vi "CSS grouping with LCS.vi"() -> ()   [LabVIEW 2014]
uses:
  <vilib>/Utility/file.llb/Read From Spreadsheet File (string).vi
  <vilib>/Utility/file.llb/Write To Spreadsheet File (string).vi
panel:
  in  "16 groups":string[][](array[string])=array2000x3[6000 elements]
  in  "8 groups":string[][](array[string])=[["0 1 0 1 0 3 0", "10", "1"], ["0 -1 1 0 1 0 3 0", "10", "1"], ["0 1 -1 0 1 0 3 0", "10", "1"], ["0 -4 1 0 1 0 3 0", "10", "1"], ["0 1 -4 0 1 0 3 0", "10", "1"], ["0 1 0 -1 1 0 3 0", "10", "1"], ["0 -1 1 0 -1 1 0 3 0", "10", "1"], ["0 1 -1 0 -1 1 0 3 0", "10", "1"], ["0 -4 1 0 -1 1 0 3 0", "10", "1"], ["0 1 -4 0 -1 1 0 3 0", "10", "1"], ["0 1 0 1 -1 0 3 0", "10", "1"], ["0 -1 1 0 1 -1 0 3 0", "10", "1"], ["0 1 -1 0 1 -1 0 3 0", "10", "1"], ["0 -4 1 0 1 -1 0 3 0", "10", "1"], ["0 1 -4 0 1 -1 0 3 0", "10", "1"], ["0 1 0 -4 1 0 3 0", "10", "1"], ["0 -1 1 0 -4 1 0 3 0", "10", "1"], ["0 1 -1 0 -4 1 0 3 0", "10", "1"], ["0 -4 1 0 -4 1 0 3 0", "10", "1"], ["0 1 -4 0 -4 1 0 3 0", "10", "1"], ["0 1 0 1 -4 0 3 0", "10", "1"], ["0 -1 1 0 1 -4 0 3 0", "10", "1"], ["0 1 -1 0 1 -4 0 3 0", "10", "1"], ["0 -4 1 0 1 -4 0 3 0", "10", "1"], ["0 1 -4 0 1 -4 0 3 0", "10", "1"], ["0 1 0 1 0 -2 3 0", "10", "1"], ["0 -1 1 0 1 0 -2 3 0", "10", "1"], ["0 1 -1 0 1 0 -2 3 0", "10", "1"], ["0 -4 1 0 1 0 -2 3 0", "10", "1"], ["0 1 -4 0 1 0 -2 3 0", "10", "1"], ["0 1 0 -1 1 0 -2 3 0", "10", "1"], ["0 -1 1 0 -1 1 0 -2 3 0", "10", "1"], ["0 1 -1 0 -1 1 0 -2 3 0", "10", "1"], ["0 -4 1 0 -1 1 0 -2 3 0", "10", "1"], ["0 1 -4 0 -1 1 0 -2 3 0", "10", "1"], ["0 1 0 1 -1 0 -2 3 0", "10", "1"], ["0 -1 1 0 1 -1 0 -2 3 0", "10", "1"], ["0 1 -1 0 1 -1 0 -2 3 0", "10", "1"], ["0 -4 1 0 1 -1 0 -2 3 0", "10", "1"], ["0 1 -4 0 1 -1 0 -2 3 0", "10", "1"], ["0 1 0 -4 1 0 -2 3 0", "10", "1"], ["0 -1 1 0 -4 1 0 -2 3 0", "10", "1"], ["0 1 -1 0 -4 1 0 -2 3 0", "10", "1"], ["0 -4 1 0 -4 1 0 -2 3 0", "10", "1"], ["0 1 -4 0 -4 1 0 -2 3 0", "10", "1"], ["0 1 0 1 -4 0 -2 3 0", "10", "1"], ["0 -1 1 0 1 -4 0 -2 3 0", "10", "1"], ["0 1 -1 0 1 -4 0 -2 3 0", "10", "1"], ["0 -4 1 0 1 -4 0 -2 3 0", "10", "1"], ["0 1 -4 0 1 -4 0 -2 3 0", "10", "1"], ["0 1 0 1 0 3 -2 0", "10", "1"], ["0 -1 1 0 1 0 3 -2 0", "10", "1"], ["0 1 -1 0 1 0 3 -2 0", "10", "1"], ["0 -4 1 0 1 0 3 -2 0", "10", "1"], ["0 1 -4 0 1 0 3 -2 0", "10", "1"], ["0 1 0 -1 1 0 3 -2 0", "10", "1"], ["0 -1 1 0 -1 1 0 3 -2 0", "10", "1"], ["0 1 -1 0 -1 1 0 3 -2 0", "10", "1"], ["0 -4 1 0 -1 1 0 3 -2 0", "10", "1"], ["0 1 -4 0 -1 1 0 3 -2 0", "10", "1"], ["0 1 0 1 -1 0 3 -2 0", "10", "1"], ["0 -1 1 0 1 -1 0 3 -2 0", "10", "1"], ["0 1 -1 0 1 -1 0 3 -2 0", "10", "1"], ["0 -4 1 0 1 -1 0 3 -2 0", "10", "1"], ["0 1 -4 0 1 -1 0 3 -2 0", "10", "1"], ["0 1 0 -4 1 0 3 -2 0", "10", "1"], ["0 -1 1 0 -4 1 0 3 -2 0", "10", "1"], ["0 1 -1 0 -4 1 0 3 -2 0", "10", "1"], ["0 -4 1 0 -4 1 0 3 -2 0", "10", "1"], ["0 1 -4 0 -4 1 0 3 -2 0", "10", "1"], ["0 1 0 1 -4 0 3 -2 0", "10", "1"], ["0 -1 1 0 1 -4 0 3 -2 0", "10", "1"], ["0 1 -1 0 1 -4 0 3 -2 0", "10", "1"], ["0 -4 1 0 1 -4 0 3 -2 0", "10", "1"], ["0 1 -4 0 1 -4 0 3 -2 0", "10", "1"], ["0 1 0 1 0 -3 3 0", "10", "1"], ["0 -1 1 0 1 0 -3 3 0", "10", "1"], ["0 1 -1 0 1 0 -3 3 0", "10", "1"], ["0 -4 1 0 1 0 -3 3 0", "10", "1"], ["0 1 -4 0 1 0 -3 3 0", "10", "1"], ["0 1 0 -1 1 0 -3 3 0", "10", "1"], ["0 -1 1 0 -1 1 0 -3 3 0", "10", "1"], ["0 1 -1 0 -1 1 0 -3 3 0", "10", "1"], ["0 -4 1 0 -1 1 0 -3 3 0", "10", "1"], ["0 1 -4 0 -1 1 0 -3 3 0", "10", "1"], ["0 1 0 1 -1 0 -3 3 0", "10", "1"], ["0 -1 1 0 1 -1 0 -3 3 0", "10", "1"], ["0 1 -1 0 1 -1 0 -3 3 0", "10", "1"], ["0 -4 1 0 1 -1 0 -3 3 0", "10", "1"], ["0 1 -4 0 1 -1 0 -3 3 0", "10", "1"], ["0 1 0 -4 1 0 -3 3 0", "10", "1"], ["0 -1 1 0 -4 1 0 -3 3 0", "10", "1"], ["0 1 -1 0 -4 1 0 -3 3 0", "10", "1"], ["0 -4 1 0 -4 1 0 -3 3 0", "10", "1"], ["0 1 -4 0 -4 1 0 -3 3 0", "10", "1"], ["0 1 0 1 -4 0 -3 3 0", "10", "1"], ["0 -1 1 0 1 -4 0 -3 3 0", "10", "1"], ["0 1 -1 0 1 -4 0 -3 3 0", "10", "1"], ["0 -4 1 0 1 -4 0 -3 3 0", "10", "1"], ["0 1 -4 0 1 -4 0 -3 3 0", "10", "1"], ["0 1 0 1 0 3 -3 0", "10", "1"], ["0 -1 1 0 1 0 3 -3 0", "10", "1"], ["0 1 -1 0 1 0 3 -3 0", "10", "1"], ["0 -4 1 0 1 0 3 -3 0", "10", "1"], ["0 1 -4 0 1 0 3 -3 0", "10", "1"], ["0 1 0 -1 1 0 3 -3 0", "10", "1"], ["0 -1 1 0 -1 1 0 3 -3 0", "10", "1"], ["0 1 -1 0 -1 1 0 3 -3 0", "10", "1"], ["0 -4 1 0 -1 1 0 3 -3 0", "10", "1"], ["0 1 -4 0 -1 1 0 3 -3 0", "10", "1"], ["0 1 0 1 -1 0 3 -3 0", "10", "1"], ["0 -1 1 0 1 -1 0 3 -3 0", "10", "1"], ["0 1 -1 0 1 -1 0 3 -3 0", "10", "1"], ["0 -4 1 0 1 -1 0 3 -3 0", "10", "1"], ["0 1 -4 0 1 -1 0 3 -3 0", "10", "1"], ["0 1 0 -4 1 0 3 -3 0", "10", "1"], ["0 -1 1 0 -4 1 0 3 -3 0", "10", "1"], ["0 1 -1 0 -4 1 0 3 -3 0", "10", "1"], ["0 -4 1 0 -4 1 0 3 -3 0", "10", "1"], ["0 1 -4 0 -4 1 0 3 -3 0", "10", "1"], ["0 1 0 1 -4 0 3 -3 0", "10", "1"], ["0 -1 1 0 1 -4 0 3 -3 0", "10", "1"], ["0 1 -1 0 1 -4 0 3 -3 0", "10", "1"], ["0 -4 1 0 1 -4 0 3 -3 0", "10", "1"], ["0 1 -4 0 1 -4 0 3 -3 0", "10", "1"], ["0 1 0 3 0 1 0", "10", "2"], ["0 -1 1 0 3 0 1 0", "10", "2"], ["0 1 -1 0 3 0 1 0", "10", "2"], ["0 -4 1 0 3 0 1 0", "10", "2"], ["0 1 -4 0 3 0 1 0", "10", "2"], ["0 1 0 -2 3 0 1 0", "10", "2"], ["0 -1 1 0 -2 3 0 1 0", "10", "2"], ["0 1 -1 0 -2 3 0 1 0", "10", "2"], ["0 -4 1 0 -2 3 0 1 0", "10", "2"], ["0 1 -4 0 -2 3 0 1 0", "10", "2"], ["0 1 0 3 -2 0 1 0", "10", "2"], ["0 -1 1 0 3 -2 0 1 0", "10", "2"], ["0 1 -1 0 3 -2 0 1 0", "10", "2"], ["0 -4 1 0 3 -2 0 1 0", "10", "2"], ["0 1 -4 0 3 -2 0 1 0", "10", "2"], ["0 1 0 -3 3 0 1 0", "10", "2"], ["0 -1 1 0 -3 3 0 1 0", "10", "2"], ["0 1 -1 0 -3 3 0 1 0", "10", "2"], ["0 -4 1 0 -3 3 0 1 0", "10", "2"], ["0 1 -4 0 -3 3 0 1 0", "10", "2"], ["0 1 0 3 -3 0 1 0", "10", "2"], ["0 -1 1 0 3 -3 0 1 0", "10", "2"], ["0 1 -1 0 3 -3 0 1 0", "10", "2"], ["0 -4 1 0 3 -3 0 1 0", "10", "2"], ["0 1 -4 0 3 -3 0 1 0", "10", "2"], ["0 1 0 3 0 -1 1 0", "10", "2"], ["0 -1 1 0 3 0 -1 1 0", "10", "2"], ["0 1 -1 0 3 0 -1 1 0", "10", "2"], ["0 -4 1 0 3 0 -1 1 0", "10", "2"], ["0 1 -4 0 3 0 -1 1 0", "10", "2"], ["0 1 0 -2 3 0 -1 1 0", "10", "2"], ["0 -1 1 0 -2 3 0 -1 1 0", "10", "2"], ["0 1 -1 0 -2 3 0 -1 1 0", "10", "2"], ["0 -4 1 0 -2 3 0 -1 1 0", "10", "2"], ["0 1 -4 0 -2 3 0 -1 1 0", "10", "2"], ["0 1 0 3 -2 0 -1 1 0", "10", "2"], ["0 -1 1 0 3 -2 0 -1 1 0", "10", "2"], ["0 1 -1 0 3 -2 0 -1 1 0", "10", "2"], ["0 -4 1 0 3 -2 0 -1 1 0", "10", "2"], ["0 1 -4 0 3 -2 0 -1 1 0", "10", "2"], ["0 1 0 -3 3 0 -1 1 0", "10", "2"], ["0 -1 1 0 -3 3 0 -1 1 0", "10", "2"], ["0 1 -1 0 -3 3 0 -1 1 0", "10", "2"], ["0 -4 1 0 -3 3 0 -1 1 0", "10", "2"], ["0 1 -4 0 -3 3 0 -1 1 0", "10", "2"], ["0 1 0 3 -3 0 -1 1 0", "10", "2"], ["0 -1 1 0 3 -3 0 -1 1 0", "10", "2"], ["0 1 -1 0 3 -3 0 -1 1 0", "10", "2"], ["0 -4 1 0 3 -3 0 -1 1 0", "10", "2"], ["0 1 -4 0 3 -3 0 -1 1 0", "10", "2"], ["0 1 0 3 0 1 -1 0", "10", "2"], ["0 -1 1 0 3 0 1 -1 0", "10", "2"], ["0 1 -1 0 3 0 1 -1 0", "10", "2"], ["0 -4 1 0 3 0 1 -1 0", "10", "2"], ["0 1 -4 0 3 0 1 -1 0", "10", "2"], ["0 1 0 -2 3 0 1 -1 0", "10", "2"], ["0 -1 1 0 -2 3 0 1 -1 0", "10", "2"], ["0 1 -1 0 -2 3 0 1 -1 0", "10", "2"], ["0 -4 1 0 -2 3 0 1 -1 0", "10", "2"], ["0 1 -4 0 -2 3 0 1 -1 0", "10", "2"], ["0 1 0 3 -2 0 1 -1 0", "10", "2"], ["0 -1 1 0 3 -2 0 1 -1 0", "10", "2"], ["0 1 -1 0 3 -2 0 1 -1 0", "10", "2"], ["0 -4 1 0 3 -2 0 1 -1 0", "10", "2"], ["0 1 -4 0 3 -2 0 1 -1 0", "10", "2"], ["0 1 0 -3 3 0 1 -1 0", "10", "2"], ["0 -1 1 0 -3 3 0 1 -1 0", "10", "2"], ["0 1 -1 0 -3 3 0 1 -1 0", "10", "2"], ["0 -4 1 0 -3 3 0 1 -1 0", "10", "2"], ["0 1 -4 0 -3 3 0 1 -1 0", "10", "2"], ["0 1 0 3 -3 0 1 -1 0", "10", "2"], ["0 -1 1 0 3 -3 0 1 -1 0", "10", "2"], ["0 1 -1 0 3 -3 0 1 -1 0", "10", "2"], ["0 -4 1 0 3 -3 0 1 -1 0", "10", "2"], ["0 1 -4 0 3 -3 0 1 -1 0", "10", "2"], ["0 1 0 3 0 -4 1 0", "10", "2"], ["0 -1 1 0 3 0 -4 1 0", "10", "2"], ["0 1 -1 0 3 0 -4 1 0", "10", "2"], ["0 -4 1 0 3 0 -4 1 0", "10", "2"], ["0 1 -4 0 3 0 -4 1 0", "10", "2"], ["0 1 0 -2 3 0 -4 1 0", "10", "2"], ["0 -1 1 0 -2 3 0 -4 1 0", "10", "2"], ["0 1 -1 0 -2 3 0 -4 1 0", "10", "2"], ["0 -4 1 0 -2 3 0 -4 1 0", "10", "2"], ["0 1 -4 0 -2 3 0 -4 1 0", "10", "2"], ["0 1 0 3 -2 0 -4 1 0", "10", "2"], ["0 -1 1 0 3 -2 0 -4 1 0", "10", "2"], ["0 1 -1 0 3 -2 0 -4 1 0", "10", "2"], ["0 -4 1 0 3 -2 0 -4 1 0", "10", "2"], ["0 1 -4 0 3 -2 0 -4 1 0", "10", "2"], ["0 1 0 -3 3 0 -4 1 0", "10", "2"], ["0 -1 1 0 -3 3 0 -4 1 0", "10", "2"], ["0 1 -1 0 -3 3 0 -4 1 0", "10", "2"], ["0 -4 1 0 -3 3 0 -4 1 0", "10", "2"], ["0 1 -4 0 -3 3 0 -4 1 0", "10", "2"], ["0 1 0 3 -3 0 -4 1 0", "10", "2"], ["0 -1 1 0 3 -3 0 -4 1 0", "10", "2"], ["0 1 -1 0 3 -3 0 -4 1 0", "10", "2"], ["0 -4 1 0 3 -3 0 -4 1 0", "10", "2"], ["0 1 -4 0 3 -3 0 -4 1 0", "10", "2"], ["0 1 0 3 0 1 -4 0", "10", "2"], ["0 -1 1 0 3 0 1 -4 0", "10", "2"], ["0 1 -1 0 3 0 1 -4 0", "10", "2"], ["0 -4 1 0 3 0 1 -4 0", "10", "2"], ["0 1 -4 0 3 0 1 -4 0", "10", "2"], ["0 1 0 -2 3 0 1 -4 0", "10", "2"], ["0 -1 1 0 -2 3 0 1 -4 0", "10", "2"], ["0 1 -1 0 -2 3 0 1 -4 0", "10", "2"], ["0 -4 1 0 -2 3 0 1 -4 0", "10", "2"], ["0 1 -4 0 -2 3 0 1 -4 0", "10", "2"], ["0 1 0 3 -2 0 1 -4 0", "10", "2"], ["0 -1 1 0 3 -2 0 1 -4 0", "10", "2"], ["0 1 -1 0 3 -2 0 1 -4 0", "10", "2"], ["0 -4 1 0 3 -2 0 1 -4 0", "10", "2"], ["0 1 -4 0 3 -2 0 1 -4 0", "10", "2"], ["0 1 0 -3 3 0 1 -4 0", "10", "2"], ["0 -1 1 0 -3 3 0 1 -4 0", "10", "2"], ["0 1 -1 0 -3 3 0 1 -4 0", "10", "2"], ["0 -4 1 0 -3 3 0 1 -4 0", "10", "2"], ["0 1 -4 0 -3 3 0 1 -4 0", "10", "2"], ["0 1 0 3 -3 0 1 -4 0", "10", "2"], ["0 -1 1 0 3 -3 0 1 -4 0", "10", "2"], ["0 1 -1 0 3 -3 0 1 -4 0", "10", "2"], ["0 -4 1 0 3 -3 0 1 -4 0", "10", "2"], ["0 1 -4 0 3 -3 0 1 -4 0", "10", "2"], ["0 3 0 3 0 1 0", "10", "3"], ["0 -2 3 0 3 0 1 0", "10", "3"], ["0 3 -2 0 3 0 1 0", "10", "3"], ["0 -3 3 0 3 0 1 0", "10", "3"], ["0 3-3 0 3 0 1 0", "10", "3"], ["0 3 0 -2 3 0 1 0", "10", "3"], ["0 -2 3 0 -2 3 0 1 0", "10", "3"], ["0 3 -2 0 -2 3 0 1 0", "10", "3"], ["0 -3 3 0 -2 3 0 1 0", "10", "3"], ["0 3-3 0 -2 3 0 1 0", "10", "3"], ["0 3 0 3 -2 0 1 0", "10", "3"], ["0 -2 3 0 3 -2 0 1 0", "10", "3"], ["0 3 -2 0 3 -2 0 1 0", "10", "3"], ["0 -3 3 0 3 -2 0 1 0", "10", "3"], ["0 3-3 0 3 -2 0 1 0", "10", "3"], ["0 3 0 -3 3 0 1 0", "10", "3"], ["0 -2 3 0 -3 3 0 1 0", "10", "3"], ["0 3 -2 0 -3 3 0 1 0", "10", "3"], ["0 -3 3 0 -3 3 0 1 0", "10", "3"], ["0 3-3 0 -3 3 0 1 0", "10", "3"], ["0 3 0 3 -3 0 1 0", "10", "3"], ["0 -2 3 0 3 -3 0 1 0", "10", "3"], ["0 3 -2 0 3 -3 0 1 0", "10", "3"], ["0 -3 3 0 3 -3 0 1 0", "10", "3"], ["0 3-3 0 3 -3 0 1 0", "10", "3"], ["0 3 0 3 0 -1 1 0", "10", "3"], ["0 -2 3 0 3 0 -1 1 0", "10", "3"], ["0 3 -2 0 3 0 -1 1 0", "10", "3"], ["0 -3 3 0 3 0 -1 1 0", "10", "3"], ["0 3-3 0 3 0 -1 1 0", "10", "3"], ["0 3 0 -2 3 0 -1 1 0", "10", "3"], ["0 -2 3 0 -2 3 0 -1 1 0", "10", "3"], ["0 3 -2 0 -2 3 0 -1 1 0", "10", "3"], ["0 -3 3 0 -2 3 0 -1 1 0", "10", "3"], ["0 3-3 0 -2 3 0 -1 1 0", "10", "3"], ["0 3 0 3 -2 0 -1 1 0", "10", "3"], ["0 -2 3 0 3 -2 0 -1 1 0", "10", "3"], ["0 3 -2 0 3 -2 0 -1 1 0", "10", "3"], ["0 -3 3 0 3 -2 0 -1 1 0", "10", "3"], ["0 3-3 0 3 -2 0 -1 1 0", "10", "3"], ["0 3 0 -3 3 0 -1 1 0", "10", "3"], ["0 -2 3 0 -3 3 0 -1 1 0", "10", "3"], ["0 3 -2 0 -3 3 0 -1 1 0", "10", "3"], ["0 -3 3 0 -3 3 0 -1 1 0", "10", "3"], ["0 3-3 0 -3 3 0 -1 1 0", "10", "3"], ["0 3 0 3 -3 0 -1 1 0", "10", "3"], ["0 -2 3 0 3 -3 0 -1 1 0", "10", "3"], ["0 3 -2 0 3 -3 0 -1 1 0", "10", "3"], ["0 -3 3 0 3 -3 0 -1 1 0", "10", "3"], ["0 3-3 0 3 -3 0 -1 1 0", "10", "3"], ["0 3 0 3 0 1 -1 0", "10", "3"], ["0 -2 3 0 3 0 1 -1 0", "10", "3"], ["0 3 -2 0 3 0 1 -1 0", "10", "3"], ["0 -3 3 0 3 0 1 -1 0", "10", "3"], ["0 3-3 0 3 0 1 -1 0", "10", "3"], ["0 3 0 -2 3 0 1 -1 0", "10", "3"], ["0 -2 3 0 -2 3 0 1 -1 0", "10", "3"], ["0 3 -2 0 -2 3 0 1 -1 0", "10", "3"], ["0 -3 3 0 -2 3 0 1 -1 0", "10", "3"], ["0 3-3 0 -2 3 0 1 -1 0", "10", "3"], ["0 3 0 3 -2 0 1 -1 0", "10", "3"], ["0 -2 3 0 3 -2 0 1 -1 0", "10", "3"], ["0 3 -2 0 3 -2 0 1 -1 0", "10", "3"], ["0 -3 3 0 3 -2 0 1 -1 0", "10", "3"], ["0 3-3 0 3 -2 0 1 -1 0", "10", "3"], ["0 3 0 -3 3 0 1 -1 0", "10", "3"], ["0 -2 3 0 -3 3 0 1 -1 0", "10", "3"], ["0 3 -2 0 -3 3 0 1 -1 0", "10", "3"], ["0 -3 3 0 -3 3 0 1 -1 0", "10", "3"], ["0 3-3 0 -3 3 0 1 -1 0", "10", "3"], ["0 3 0 3 -3 0 1 -1 0", "10", "3"], ["0 -2 3 0 3 -3 0 1 -1 0", "10", "3"], ["0 3 -2 0 3 -3 0 1 -1 0", "10", "3"], ["0 -3 3 0 3 -3 0 1 -1 0", "10", "3"], ["0 3-3 0 3 -3 0 1 -1 0", "10", "3"], ["0 3 0 3 0 -4 1 0", "10", "3"], ["0 -2 3 0 3 0 -4 1 0", "10", "3"], ["0 3 -2 0 3 0 -4 1 0", "10", "3"], ["0 -3 3 0 3 0 -4 1 0", "10", "3"], ["0 3-3 0 3 0 -4 1 0", "10", "3"], ["0 3 0 -2 3 0 -4 1 0", "10", "3"], ["0 -2 3 0 -2 3 0 -4 1 0", "10", "3"], ["0 3 -2 0 -2 3 0 -4 1 0", "10", "3"], ["0 -3 3 0 -2 3 0 -4 1 0", "10", "3"], ["0 3-3 0 -2 3 0 -4 1 0", "10", "3"], ["0 3 0 3 -2 0 -4 1 0", "10", "3"], ["0 -2 3 0 3 -2 0 -4 1 0", "10", "3"], ["0 3 -2 0 3 -2 0 -4 1 0", "10", "3"], ["0 -3 3 0 3 -2 0 -4 1 0", "10", "3"], ["0 3-3 0 3 -2 0 -4 1 0", "10", "3"], ["0 3 0 -3 3 0 -4 1 0", "10", "3"], ["0 -2 3 0 -3 3 0 -4 1 0", "10", "3"], ["0 3 -2 0 -3 3 0 -4 1 0", "10", "3"], ["0 -3 3 0 -3 3 0 -4 1 0", "10", "3"], ["0 3-3 0 -3 3 0 -4 1 0", "10", "3"], ["0 3 0 3 -3 0 -4 1 0", "10", "3"], ["0 -2 3 0 3 -3 0 -4 1 0", "10", "3"], ["0 3 -2 0 3 -3 0 -4 1 0", "10", "3"], ["0 -3 3 0 3 -3 0 -4 1 0", "10", "3"], ["0 3-3 0 3 -3 0 -4 1 0", "10", "3"], ["0 3 0 3 0 1 -4 0", "10", "3"], ["0 -2 3 0 3 0 1 -4 0", "10", "3"], ["0 3 -2 0 3 0 1 -4 0", "10", "3"], ["0 -3 3 0 3 0 1 -4 0", "10", "3"], ["0 3-3 0 3 0 1 -4 0", "10", "3"], ["0 3 0 -2 3 0 1 -4 0", "10", "3"], ["0 -2 3 0 -2 3 0 1 -4 0", "10", "3"], ["0 3 -2 0 -2 3 0 1 -4 0", "10", "3"], ["0 -3 3 0 -2 3 0 1 -4 0", "10", "3"], ["0 3-3 0 -2 3 0 1 -4 0", "10", "3"], ["0 3 0 3 -2 0 1 -4 0", "10", "3"], ["0 -2 3 0 3 -2 0 1 -4 0", "10", "3"], ["0 3 -2 0 3 -2 0 1 -4 0", "10", "3"], ["0 -3 3 0 3 -2 0 1 -4 0", "10", "3"], ["0 3-3 0 3 -2 0 1 -4 0", "10", "3"], ["0 3 0 -3 3 0 1 -4 0", "10", "3"], ["0 -2 3 0 -3 3 0 1 -4 0", "10", "3"], ["0 3 -2 0 -3 3 0 1 -4 0", "10", "3"], ["0 -3 3 0 -3 3 0 1 -4 0", "10", "3"], ["0 3-3 0 -3 3 0 1 -4 0", "10", "3"], ["0 3 0 3 -3 0 1 -4 0", "10", "3"], ["0 -2 3 0 3 -3 0 1 -4 0", "10", "3"], ["0 3 -2 0 3 -3 0 1 -4 0", "10", "3"], ["0 -3 3 0 3 -3 0 1 -4 0", "10", "3"], ["0 3-3 0 3 -3 0 1 -4 0", "10", "3"], ["0 3 0 1 0 3 0", "10", "4"], ["0 -2 3 0 1 0 3 0", "10", "4"], ["0 3 -2 0 1 0 3 0", "10", "4"], ["0 -3 3 0 1 0 3 0", "10", "4"], ["0 3-3 0 1 0 3 0", "10", "4"], ["0 3 0 -1 1 0 3 0", "10", "4"], ["0 -2 3 0 -1 1 0 3 0", "10", "4"], ["0 3 -2 0 -1 1 0 3 0", "10", "4"], ["0 -3 3 0 -1 1 0 3 0", "10", "4"], ["0 3-3 0 -1 1 0 3 0", "10", "4"], ["0 3 0 1 -1 0 3 0", "10", "4"], ["0 -2 3 0 1 -1 0 3 0", "10", "4"], ["0 3 -2 0 1 -1 0 3 0", "10", "4"], ["0 -3 3 0 1 -1 0 3 0", "10", "4"], ["0 3-3 0 1 -1 0 3 0", "10", "4"], ["0 3 0 -4 1 0 3 0", "10", "4"], ["0 -2 3 0 -4 1 0 3 0", "10", "4"], ["0 3 -2 0 -4 1 0 3 0", "10", "4"], ["0 -3 3 0 -4 1 0 3 0", "10", "4"], ["0 3-3 0 -4 1 0 3 0", "10", "4"], ["0 3 0 1 -4 0 3 0", "10", "4"], ["0 -2 3 0 1 -4 0 3 0", "10", "4"], ["0 3 -2 0 1 -4 0 3 0", "10", "4"], ["0 -3 3 0 1 -4 0 3 0", "10", "4"], ["0 3-3 0 1 -4 0 3 0", "10", "4"], ["0 3 0 1 0 -2 3 0", "10", "4"], ["0 -2 3 0 1 0 -2 3 0", "10", "4"], ["0 3 -2 0 1 0 -2 3 0", "10", "4"], ["0 -3 3 0 1 0 -2 3 0", "10", "4"], ["0 3-3 0 1 0 -2 3 0", "10", "4"], ["0 3 0 -1 1 0 -2 3 0", "10", "4"], ["0 -2 3 0 -1 1 0 -2 3 0", "10", "4"], ["0 3 -2 0 -1 1 0 -2 3 0", "10", "4"], ["0 -3 3 0 -1 1 0 -2 3 0", "10", "4"], ["0 3-3 0 -1 1 0 -2 3 0", "10", "4"], ["0 3 0 1 -1 0 -2 3 0", "10", "4"], ["0 -2 3 0 1 -1 0 -2 3 0", "10", "4"], ["0 3 -2 0 1 -1 0 -2 3 0", "10", "4"], ["0 -3 3 0 1 -1 0 -2 3 0", "10", "4"], ["0 3-3 0 1 -1 0 -2 3 0", "10", "4"], ["0 3 0 -4 1 0 -2 3 0", "10", "4"], ["0 -2 3 0 -4 1 0 -2 3 0", "10", "4"], ["0 3 -2 0 -4 1 0 -2 3 0", "10", "4"], ["0 -3 3 0 -4 1 0 -2 3 0", "10", "4"], ["0 3-3 0 -4 1 0 -2 3 0", "10", "4"], ["0 3 0 1 -4 0 -2 3 0", "10", "4"], ["0 -2 3 0 1 -4 0 -2 3 0", "10", "4"], ["0 3 -2 0 1 -4 0 -2 3 0", "10", "4"], ["0 -3 3 0 1 -4 0 -2 3 0", "10", "4"], ["0 3-3 0 1 -4 0 -2 3 0", "10", "4"], ["0 3 0 1 0 3 -2 0", "10", "4"], ["0 -2 3 0 1 0 3 -2 0", "10", "4"], ["0 3 -2 0 1 0 3 -2 0", "10", "4"], ["0 -3 3 0 1 0 3 -2 0", "10", "4"], ["0 3-3 0 1 0 3 -2 0", "10", "4"], ["0 3 0 -1 1 0 3 -2 0", "10", "4"], ["0 -2 3 0 -1 1 0 3 -2 0", "10", "4"], ["0 3 -2 0 -1 1 0 3 -2 0", "10", "4"], ["0 -3 3 0 -1 1 0 3 -2 0", "10", "4"], ["0 3-3 0 -1 1 0 3 -2 0", "10", "4"], ["0 3 0 1 -1 0 3 -2 0", "10", "4"], ["0 -2 3 0 1 -1 0 3 -2 0", "10", "4"], ["0 3 -2 0 1 -1 0 3 -2 0", "10", "4"], ["0 -3 3 0 1 -1 0 3 -2 0", "10", "4"], ["0 3-3 0 1 -1 0 3 -2 0", "10", "4"], ["0 3 0 -4 1 0 3 -2 0", "10", "4"], ["0 -2 3 0 -4 1 0 3 -2 0", "10", "4"], ["0 3 -2 0 -4 1 0 3 -2 0", "10", "4"], ["0 -3 3 0 -4 1 0 3 -2 0", "10", "4"], ["0 3-3 0 -4 1 0 3 -2 0", "10", "4"], ["0 3 0 1 -4 0 3 -2 0", "10", "4"], ["0 -2 3 0 1 -4 0 3 -2 0", "10", "4"], ["0 3 -2 0 1 -4 0 3 -2 0", "10", "4"], ["0 -3 3 0 1 -4 0 3 -2 0", "10", "4"], ["0 3-3 0 1 -4 0 3 -2 0", "10", "4"], ["0 3 0 1 0 -3 3 0", "10", "4"], ["0 -2 3 0 1 0 -3 3 0", "10", "4"], ["0 3 -2 0 1 0 -3 3 0", "10", "4"], ["0 -3 3 0 1 0 -3 3 0", "10", "4"], ["0 3-3 0 1 0 -3 3 0", "10", "4"], ["0 3 0 -1 1 0 -3 3 0", "10", "4"], ["0 -2 3 0 -1 1 0 -3 3 0", "10", "4"], ["0 3 -2 0 -1 1 0 -3 3 0", "10", "4"], ["0 -3 3 0 -1 1 0 -3 3 0", "10", "4"], ["0 3-3 0 -1 1 0 -3 3 0", "10", "4"], ["0 3 0 1 -1 0 -3 3 0", "10", "4"], ["0 -2 3 0 1 -1 0 -3 3 0", "10", "4"], ["0 3 -2 0 1 -1 0 -3 3 0", "10", "4"], ["0 -3 3 0 1 -1 0 -3 3 0", "10", "4"], ["0 3-3 0 1 -1 0 -3 3 0", "10", "4"], ["0 3 0 -4 1 0 -3 3 0", "10", "4"], ["0 -2 3 0 -4 1 0 -3 3 0", "10", "4"], ["0 3 -2 0 -4 1 0 -3 3 0", "10", "4"], ["0 -3 3 0 -4 1 0 -3 3 0", "10", "4"], ["0 3-3 0 -4 1 0 -3 3 0", "10", "4"], ["0 3 0 1 -4 0 -3 3 0", "10", "4"], ["0 -2 3 0 1 -4 0 -3 3 0", "10", "4"], ["0 3 -2 0 1 -4 0 -3 3 0", "10", "4"], ["0 -3 3 0 1 -4 0 -3 3 0", "10", "4"], ["0 3-3 0 1 -4 0 -3 3 0", "10", "4"], ["0 3 0 1 0 3 -3 0", "10", "4"], ["0 -2 3 0 1 0 3 -3 0", "10", "4"], ["0 3 -2 0 1 0 3 -3 0", "10", "4"], ["0 -3 3 0 1 0 3 -3 0", "10", "4"], ["0 3-3 0 1 0 3 -3 0", "10", "4"], ["0 3 0 -1 1 0 3 -3 0", "10", "4"], ["0 -2 3 0 -1 1 0 3 -3 0", "10", "4"], ["0 3 -2 0 -1 1 0 3 -3 0", "10", "4"], ["0 -3 3 0 -1 1 0 3 -3 0", "10", "4"], ["0 3-3 0 -1 1 0 3 -3 0", "10", "4"], ["0 3 0 1 -1 0 3 -3 0", "10", "4"], ["0 -2 3 0 1 -1 0 3 -3 0", "10", "4"], ["0 3 -2 0 1 -1 0 3 -3 0", "10", "4"], ["0 -3 3 0 1 -1 0 3 -3 0", "10", "4"], ["0 3-3 0 1 -1 0 3 -3 0", "10", "4"], ["0 3 0 -4 1 0 3 -3 0", "10", "4"], ["0 -2 3 0 -4 1 0 3 -3 0", "10", "4"], ["0 3 -2 0 -4 1 0 3 -3 0", "10", "4"], ["0 -3 3 0 -4 1 0 3 -3 0", "10", "4"], ["0 3-3 0 -4 1 0 3 -3 0", "10", "4"], ["0 3 0 1 -4 0 3 -3 0", "10", "4"], ["0 -2 3 0 1 -4 0 3 -3 0", "10", "4"], ["0 3 -2 0 1 -4 0 3 -3 0", "10", "4"], ["0 -3 3 0 1 -4 0 3 -3 0", "10", "4"], ["0 3-3 0 1 -4 0 3 -3 0", "10", "4"], ["0 2 0 2 0 4 0", "10", "5"], ["0 -1 2 0 2 0 4 0", "10", "5"], ["0 2 -1 0 2 0 4 0", "10", "5"], ["0 -2 2 0 2 0 4 0", "10", "5"], ["0 2 -2 0 2 0 4 0", "10", "5"], ["0 2 0 -1 2 0 4 0", "10", "5"], ["0 -1 2 0 -1 2 0 4 0", "10", "5"], ["0 2 -1 0 -1 2 0 4 0", "10", "5"], ["0 -2 2 0 -1 2 0 4 0", "10", "5"], ["0 2 -2 0 -1 2 0 4 0", "10", "5"], ["0 2 0 2 -1 0 4 0", "10", "5"], ["0 -1 2 0 2 -1 0 4 0", "10", "5"], ["0 2 -1 0 2 -1 0 4 0", "10", "5"], ["0 -2 2 0 2 -1 0 4 0", "10", "5"], ["0 2 -2 0 2 -1 0 4 0", "10", "5"], ["0 2 0 -2 2 0 4 0", "10", "5"], ["0 -1 2 0 -2 2 0 4 0", "10", "5"], ["0 2 -1 0 -2 2 0 4 0", "10", "5"], ["0 -2 2 0 -2 2 0 4 0", "10", "5"], ["0 2 -2 0 -2 2 0 4 0", "10", "5"], ["0 2 0 2 -2 0 4 0", "10", "5"], ["0 -1 2 0 2 -2 0 4 0", "10", "5"], ["0 2 -1 0 2 -2 0 4 0", "10", "5"], ["0 -2 2 0 2 -2 0 4 0", "10", "5"], ["0 2 -2 0 2 -2 0 4 0", "10", "5"], ["0 2 0 2 0 -3 4 0", "10", "5"], ["0 -1 2 0 2 0 -3 4 0", "10", "5"], ["0 2 -1 0 2 0 -3 4 0", "10", "5"], ["0 -2 2 0 2 0 -3 4 0", "10", "5"], ["0 2 -2 0 2 0 -3 4 0", "10", "5"], ["0 2 0 -1 2 0 -3 4 0", "10", "5"], ["0 -1 2 0 -1 2 0 -3 4 0", "10", "5"], ["0 2 -1 0 -1 2 0 -3 4 0", "10", "5"], ["0 -2 2 0 -1 2 0 -3 4 0", "10", "5"], ["0 2 -2 0 -1 2 0 -3 4 0", "10", "5"], ["0 2 0 2 -1 0 -3 4 0", "10", "5"], ["0 -1 2 0 2 -1 0 -3 4 0", "10", "5"], ["0 2 -1 0 2 -1 0 -3 4 0", "10", "5"], ["0 -2 2 0 2 -1 0 -3 4 0", "10", "5"], ["0 2 -2 0 2 -1 0 -3 4 0", "10", "5"], ["0 2 0 -2 2 0 -3 4 0", "10", "5"], ["0 -1 2 0 -2 2 0 -3 4 0", "10", "5"], ["0 2 -1 0 -2 2 0 -3 4 0", "10", "5"], ["0 -2 2 0 -2 2 0 -3 4 0", "10", "5"], ["0 2 -2 0 -2 2 0 -3 4 0", "10", "5"], ["0 2 0 2 -2 0 -3 4 0", "10", "5"], ["0 -1 2 0 2 -2 0 -3 4 0", "10", "5"], ["0 2 -1 0 2 -2 0 -3 4 0", "10", "5"], ["0 -2 2 0 2 -2 0 -3 4 0", "10", "5"], ["0 2 -2 0 2 -2 0 -3 4 0", "10", "5"], ["0 2 0 2 0 4 -3 0", "10", "5"], ["0 -1 2 0 2 0 4 -3 0", "10", "5"], ["0 2 -1 0 2 0 4 -3 0", "10", "5"], ["0 -2 2 0 2 0 4 -3 0", "10", "5"], ["0 2 -2 0 2 0 4 -3 0", "10", "5"], ["0 2 0 -1 2 0 4 -3 0", "10", "5"], ["0 -1 2 0 -1 2 0 4 -3 0", "10", "5"], ["0 2 -1 0 -1 2 0 4 -3 0", "10", "5"], ["0 -2 2 0 -1 2 0 4 -3 0", "10", "5"], ["0 2 -2 0 -1 2 0 4 -3 0", "10", "5"], ["0 2 0 2 -1 0 4 -3 0", "10", "5"], ["0 -1 2 0 2 -1 0 4 -3 0", "10", "5"], ["0 2 -1 0 2 -1 0 4 -3 0", "10", "5"], ["0 -2 2 0 2 -1 0 4 -3 0", "10", "5"], ["0 2 -2 0 2 -1 0 4 -3 0", "10", "5"], ["0 2 0 -2 2 0 4 -3 0", "10", "5"], ["0 -1 2 0 -2 2 0 4 -3 0", "10", "5"], ["0 2 -1 0 -2 2 0 4 -3 0", "10", "5"], ["0 -2 2 0 -2 2 0 4 -3 0", "10", "5"], ["0 2 -2 0 -2 2 0 4 -3 0", "10", "5"], ["0 2 0 2 -2 0 4 -3 0", "10", "5"], ["0 -1 2 0 2 -2 0 4 -3 0", "10", "5"], ["0 2 -1 0 2 -2 0 4 -3 0", "10", "5"], ["0 -2 2 0 2 -2 0 4 -3 0", "10", "5"], ["0 2 -2 0 2 -2 0 4 -3 0", "10", "5"], ["0 2 0 2 0 -4 4 0", "10", "5"], ["0 -1 2 0 2 0 -4 4 0", "10", "5"], ["0 2 -1 0 2 0 -4 4 0", "10", "5"], ["0 -2 2 0 2 0 -4 4 0", "10", "5"], ["0 2 -2 0 2 0 -4 4 0", "10", "5"], ["0 2 0 -1 2 0 -4 4 0", "10", "5"], ["0 -1 2 0 -1 2 0 -4 4 0", "10", "5"], ["0 2 -1 0 -1 2 0 -4 4 0", "10", "5"], ["0 -2 2 0 -1 2 0 -4 4 0", "10", "5"], ["0 2 -2 0 -1 2 0 -4 4 0", "10", "5"], ["0 2 0 2 -1 0 -4 4 0", "10", "5"], ["0 -1 2 0 2 -1 0 -4 4 0", "10", "5"], ["0 2 -1 0 2 -1 0 -4 4 0", "10", "5"], ["0 -2 2 0 2 -1 0 -4 4 0", "10", "5"], ["0 2 -2 0 2 -1 0 -4 4 0", "10", "5"], ["0 2 0 -2 2 0 -4 4 0", "10", "5"], ["0 -1 2 0 -2 2 0 -4 4 0", "10", "5"], ["0 2 -1 0 -2 2 0 -4 4 0", "10", "5"], ["0 -2 2 0 -2 2 0 -4 4 0", "10", "5"], ["0 2 -2 0 -2 2 0 -4 4 0", "10", "5"], ["0 2 0 2 -2 0 -4 4 0", "10", "5"], ["0 -1 2 0 2 -2 0 -4 4 0", "10", "5"], ["0 2 -1 0 2 -2 0 -4 4 0", "10", "5"], ["0 -2 2 0 2 -2 0 -4 4 0", "10", "5"], ["0 2 -2 0 2 -2 0 -4 4 0", "10", "5"], ["0 2 0 2 0 4 -4 0", "10", "5"], ["0 -1 2 0 2 0 4 -4 0", "10", "5"], ["0 2 -1 0 2 0 4 -4 0", "10", "5"], ["0 -2 2 0 2 0 4 -4 0", "10", "5"], ["0 2 -2 0 2 0 4 -4 0", "10", "5"], ["0 2 0 -1 2 0 4 -4 0", "10", "5"], ["0 -1 2 0 -1 2 0 4 -4 0", "10", "5"], ["0 2 -1 0 -1 2 0 4 -4 0", "10", "5"], ["0 -2 2 0 -1 2 0 4 -4 0", "10", "5"], ["0 2 -2 0 -1 2 0 4 -4 0", "10", "5"], ["0 2 0 2 -1 0 4 -4 0", "10", "5"], ["0 -1 2 0 2 -1 0 4 -4 0", "10", "5"], ["0 2 -1 0 2 -1 0 4 -4 0", "10", "5"], ["0 -2 2 0 2 -1 0 4 -4 0", "10", "5"], ["0 2 -2 0 2 -1 0 4 -4 0", "10", "5"], ["0 2 0 -2 2 0 4 -4 0", "10", "5"], ["0 -1 2 0 -2 2 0 4 -4 0", "10", "5"], ["0 2 -1 0 -2 2 0 4 -4 0", "10", "5"], ["0 -2 2 0 -2 2 0 4 -4 0", "10", "5"], ["0 2 -2 0 -2 2 0 4 -4 0", "10", "5"], ["0 2 0 2 -2 0 4 -4 0", "10", "5"], ["0 -1 2 0 2 -2 0 4 -4 0", "10", "5"], ["0 2 -1 0 2 -2 0 4 -4 0", "10", "5"], ["0 -2 2 0 2 -2 0 4 -4 0", "10", "5"], ["0 2 -2 0 2 -2 0 4 -4 0", "10", "5"], ["0 2 0 4 0 2 0", "10", "6"], ["0 -1 2 0 4 0 2 0", "10", "6"], ["0 2 -1 0 4 0 2 0", "10", "6"], ["0 -2 2 0 4 0 2 0", "10", "6"], ["0 2 -2 0 4 0 2 0", "10", "6"], ["0 2 0 -3 4 0 2 0", "10", "6"], ["0 -1 2 0 -3 4 0 2 0", "10", "6"], ["0 2 -1 0 -3 4 0 2 0", "10", "6"], ["0 -2 2 0 -3 4 0 2 0", "10", "6"], ["0 2 -2 0 -3 4 0 2 0", "10", "6"], ["0 2 0 4 -3 0 2 0", "10", "6"], ["0 -1 2 0 4 -3 0 2 0", "10", "6"], ["0 2 -1 0 4 -3 0 2 0", "10", "6"], ["0 -2 2 0 4 -3 0 2 0", "10", "6"], ["0 2 -2 0 4 -3 0 2 0", "10", "6"], ["0 2 0 -4 4 0 2 0", "10", "6"], ["0 -1 2 0 -4 4 0 2 0", "10", "6"], ["0 2 -1 0 -4 4 0 2 0", "10", "6"], ["0 -2 2 0 -4 4 0 2 0", "10", "6"], ["0 2 -2 0 -4 4 0 2 0", "10", "6"], ["0 2 0 4 -4 0 2 0", "10", "6"], ["0 -1 2 0 4 -4 0 2 0", "10", "6"], ["0 2 -1 0 4 -4 0 2 0", "10", "6"], ["0 -2 2 0 4 -4 0 2 0", "10", "6"], ["0 2 -2 0 4 -4 0 2 0", "10", "6"], ["0 2 0 4 0 -1 2 0", "10", "6"], ["0 -1 2 0 4 0 -1 2 0", "10", "6"], ["0 2 -1 0 4 0 -1 2 0", "10", "6"], ["0 -2 2 0 4 0 -1 2 0", "10", "6"], ["0 2 -2 0 4 0 -1 2 0", "10", "6"], ["0 2 0 -3 4 0 -1 2 0", "10", "6"], ["0 -1 2 0 -3 4 0 -1 2 0", "10", "6"], ["0 2 -1 0 -3 4 0 -1 2 0", "10", "6"], ["0 -2 2 0 -3 4 0 -1 2 0", "10", "6"], ["0 2 -2 0 -3 4 0 -1 2 0", "10", "6"], ["0 2 0 4 -3 0 -1 2 0", "10", "6"], ["0 -1 2 0 4 -3 0 -1 2 0", "10", "6"], ["0 2 -1 0 4 -3 0 -1 2 0", "10", "6"], ["0 -2 2 0 4 -3 0 -1 2 0", "10", "6"], ["0 2 -2 0 4 -3 0 -1 2 0", "10", "6"], ["0 2 0 -4 4 0 -1 2 0", "10", "6"], ["0 -1 2 0 -4 4 0 -1 2 0", "10", "6"], ["0 2 -1 0 -4 4 0 -1 2 0", "10", "6"], ["0 -2 2 0 -4 4 0 -1 2 0", "10", "6"], ["0 2 -2 0 -4 4 0 -1 2 0", "10", "6"], ["0 2 0 4 -4 0 -1 2 0", "10", "6"], ["0 -1 2 0 4 -4 0 -1 2 0", "10", "6"], ["0 2 -1 0 4 -4 0 -1 2 0", "10", "6"], ["0 -2 2 0 4 -4 0 -1 2 0", "10", "6"], ["0 2 -2 0 4 -4 0 -1 2 0", "10", "6"], ["0 2 0 4 0 2 -1 0", "10", "6"], ["0 -1 2 0 4 0 2 -1 0", "10", "6"], ["0 2 -1 0 4 0 2 -1 0", "10", "6"], ["0 -2 2 0 4 0 2 -1 0", "10", "6"], ["0 2 -2 0 4 0 2 -1 0", "10", "6"], ["0 2 0 -3 4 0 2 -1 0", "10", "6"], ["0 -1 2 0 -3 4 0 2 -1 0", "10", "6"], ["0 2 -1 0 -3 4 0 2 -1 0", "10", "6"], ["0 -2 2 0 -3 4 0 2 -1 0", "10", "6"], ["0 2 -2 0 -3 4 0 2 -1 0", "10", "6"], ["0 2 0 4 -3 0 2 -1 0", "10", "6"], ["0 -1 2 0 4 -3 0 2 -1 0", "10", "6"], ["0 2 -1 0 4 -3 0 2 -1 0", "10", "6"], ["0 -2 2 0 4 -3 0 2 -1 0", "10", "6"], ["0 2 -2 0 4 -3 0 2 -1 0", "10", "6"], ["0 2 0 -4 4 0 2 -1 0", "10", "6"], ["0 -1 2 0 -4 4 0 2 -1 0", "10", "6"], ["0 2 -1 0 -4 4 0 2 -1 0", "10", "6"], ["0 -2 2 0 -4 4 0 2 -1 0", "10", "6"], ["0 2 -2 0 -4 4 0 2 -1 0", "10", "6"], ["0 2 0 4 -4 0 2 -1 0", "10", "6"], ["0 -1 2 0 4 -4 0 2 -1 0", "10", "6"], ["0 2 -1 0 4 -4 0 2 -1 0", "10", "6"], ["0 -2 2 0 4 -4 0 2 -1 0", "10", "6"], ["0 2 -2 0 4 -4 0 2 -1 0", "10", "6"], ["0 2 0 4 0 -2 2 0", "10", "6"], ["0 -1 2 0 4 0 -2 2 0", "10", "6"], ["0 2 -1 0 4 0 -2 2 0", "10", "6"], ["0 -2 2 0 4 0 -2 2 0", "10", "6"], ["0 2 -2 0 4 0 -2 2 0", "10", "6"], ["0 2 0 -3 4 0 -2 2 0", "10", "6"], ["0 -1 2 0 -3 4 0 -2 2 0", "10", "6"], ["0 2 -1 0 -3 4 0 -2 2 0", "10", "6"], ["0 -2 2 0 -3 4 0 -2 2 0", "10", "6"], ["0 2 -2 0 -3 4 0 -2 2 0", "10", "6"], ["0 2 0 4 -3 0 -2 2 0", "10", "6"], ["0 -1 2 0 4 -3 0 -2 2 0", "10", "6"], ["0 2 -1 0 4 -3 0 -2 2 0", "10", "6"], ["0 -2 2 0 4 -3 0 -2 2 0", "10", "6"], ["0 2 -2 0 4 -3 0 -2 2 0", "10", "6"], ["0 2 0 -4 4 0 -2 2 0", "10", "6"], ["0 -1 2 0 -4 4 0 -2 2 0", "10", "6"], ["0 2 -1 0 -4 4 0 -2 2 0", "10", "6"], ["0 -2 2 0 -4 4 0 -2 2 0", "10", "6"], ["0 2 -2 0 -4 4 0 -2 2 0", "10", "6"], ["0 2 0 4 -4 0 -2 2 0", "10", "6"], ["0 -1 2 0 4 -4 0 -2 2 0", "10", "6"], ["0 2 -1 0 4 -4 0 -2 2 0", "10", "6"], ["0 -2 2 0 4 -4 0 -2 2 0", "10", "6"], ["0 2 -2 0 4 -4 0 -2 2 0", "10", "6"], ["0 2 0 4 0 2 -2 0", "10", "6"], ["0 -1 2 0 4 0 2 -2 0", "10", "6"], ["0 2 -1 0 4 0 2 -2 0", "10", "6"], ["0 -2 2 0 4 0 2 -2 0", "10", "6"], ["0 2 -2 0 4 0 2 -2 0", "10", "6"], ["0 2 0 -3 4 0 2 -2 0", "10", "6"], ["0 -1 2 0 -3 4 0 2 -2 0", "10", "6"], ["0 2 -1 0 -3 4 0 2 -2 0", "10", "6"], ["0 -2 2 0 -3 4 0 2 -2 0", "10", "6"], ["0 2 -2 0 -3 4 0 2 -2 0", "10", "6"], ["0 2 0 4 -3 0 2 -2 0", "10", "6"], ["0 -1 2 0 4 -3 0 2 -2 0", "10", "6"], ["0 2 -1 0 4 -3 0 2 -2 0", "10", "6"], ["0 -2 2 0 4 -3 0 2 -2 0", "10", "6"], ["0 2 -2 0 4 -3 0 2 -2 0", "10", "6"], ["0 2 0 -4 4 0 2 -2 0", "10", "6"], ["0 -1 2 0 -4 4 0 2 -2 0", "10", "6"], ["0 2 -1 0 -4 4 0 2 -2 0", "10", "6"], ["0 -2 2 0 -4 4 0 2 -2 0", "10", "6"], ["0 2 -2 0 -4 4 0 2 -2 0", "10", "6"], ["0 2 0 4 -4 0 2 -2 0", "10", "6"], ["0 -1 2 0 4 -4 0 2 -2 0", "10", "6"], ["0 2 -1 0 4 -4 0 2 -2 0", "10", "6"], ["0 -2 2 0 4 -4 0 2 -2 0", "10", "6"], ["0 2 -2 0 4 -4 0 2 -2 0", "10", "6"], ["0 4 0 4 0 2 0", "10", "7"], ["0 -3 4 0 4 0 2 0", "10", "7"], ["0 4 -3 0 4 0 2 0", "10", "7"], ["0 -4 4 0 4 0 2 0", "10", "7"], ["0 4 -4 0 4 0 2 0", "10", "7"], ["0 4 0 -3 4 0 2 0", "10", "7"], ["0 -3 4 0 -3 4 0 2 0", "10", "7"], ["0 4 -3 0 -3 4 0 2 0", "10", "7"], ["0 -4 4 0 -3 4 0 2 0", "10", "7"], ["0 4 -4 0 -3 4 0 2 0", "10", "7"], ["0 4 0 4 -3 0 2 0", "10", "7"], ["0 -3 4 0 4 -3 0 2 0", "10", "7"], ["0 4 -3 0 4 -3 0 2 0", "10", "7"], ["0 -4 4 0 4 -3 0 2 0", "10", "7"], ["0 4 -4 0 4 -3 0 2 0", "10", "7"], ["0 4 0 -4 4 0 2 0", "10", "7"], ["0 -3 4 0 -4 4 0 2 0", "10", "7"], ["0 4 -3 0 -4 4 0 2 0", "10", "7"], ["0 -4 4 0 -4 4 0 2 0", "10", "7"], ["0 4 -4 0 -4 4 0 2 0", "10", "7"], ["0 4 0 4 -4 0 2 0", "10", "7"], ["0 -3 4 0 4 -4 0 2 0", "10", "7"], ["0 4 -3 0 4 -4 0 2 0", "10", "7"], ["0 -4 4 0 4 -4 0 2 0", "10", "7"], ["0 4 -4 0 4 -4 0 2 0", "10", "7"], ["0 4 0 4 0 -1 2 0", "10", "7"], ["0 -3 4 0 4 0 -1 2 0", "10", "7"], ["0 4 -3 0 4 0 -1 2 0", "10", "7"], ["0 -4 4 0 4 0 -1 2 0", "10", "7"], ["0 4 -4 0 4 0 -1 2 0", "10", "7"], ["0 4 0 -3 4 0 -1 2 0", "10", "7"], ["0 -3 4 0 -3 4 0 -1 2 0", "10", "7"], ["0 4 -3 0 -3 4 0 -1 2 0", "10", "7"], ["0 -4 4 0 -3 4 0 -1 2 0", "10", "7"], ["0 4 -4 0 -3 4 0 -1 2 0", "10", "7"], ["0 4 0 4 -3 0 -1 2 0", "10", "7"], ["0 -3 4 0 4 -3 0 -1 2 0", "10", "7"], ["0 4 -3 0 4 -3 0 -1 2 0", "10", "7"], ["0 -4 4 0 4 -3 0 -1 2 0", "10", "7"], ["0 4 -4 0 4 -3 0 -1 2 0", "10", "7"], ["0 4 0 -4 4 0 -1 2 0", "10", "7"], ["0 -3 4 0 -4 4 0 -1 2 0", "10", "7"], ["0 4 -3 0 -4 4 0 -1 2 0", "10", "7"], ["0 -4 4 0 -4 4 0 -1 2 0", "10", "7"], ["0 4 -4 0 -4 4 0 -1 2 0", "10", "7"], ["0 4 0 4 -4 0 -1 2 0", "10", "7"], ["0 -3 4 0 4 -4 0 -1 2 0", "10", "7"], ["0 4 -3 0 4 -4 0 -1 2 0", "10", "7"], ["0 -4 4 0 4 -4 0 -1 2 0", "10", "7"], ["0 4 -4 0 4 -4 0 -1 2 0", "10", "7"], ["0 4 0 4 0 2 -1 0", "10", "7"], ["0 -3 4 0 4 0 2 -1 0", "10", "7"], ["0 4 -3 0 4 0 2 -1 0", "10", "7"], ["0 -4 4 0 4 0 2 -1 0", "10", "7"], ["0 4 -4 0 4 0 2 -1 0", "10", "7"], ["0 4 0 -3 4 0 2 -1 0", "10", "7"], ["0 -3 4 0 -3 4 0 2 -1 0", "10", "7"], ["0 4 -3 0 -3 4 0 2 -1 0", "10", "7"], ["0 -4 4 0 -3 4 0 2 -1 0", "10", "7"], ["0 4 -4 0 -3 4 0 2 -1 0", "10", "7"], ["0 4 0 4 -3 0 2 -1 0", "10", "7"], ["0 -3 4 0 4 -3 0 2 -1 0", "10", "7"], ["0 4 -3 0 4 -3 0 2 -1 0", "10", "7"], ["0 -4 4 0 4 -3 0 2 -1 0", "10", "7"], ["0 4 -4 0 4 -3 0 2 -1 0", "10", "7"], ["0 4 0 -4 4 0 2 -1 0", "10", "7"], ["0 -3 4 0 -4 4 0 2 -1 0", "10", "7"], ["0 4 -3 0 -4 4 0 2 -1 0", "10", "7"], ["0 -4 4 0 -4 4 0 2 -1 0", "10", "7"], ["0 4 -4 0 -4 4 0 2 -1 0", "10", "7"], ["0 4 0 4 -4 0 2 -1 0", "10", "7"], ["0 -3 4 0 4 -4 0 2 -1 0", "10", "7"], ["0 4 -3 0 4 -4 0 2 -1 0", "10", "7"], ["0 -4 4 0 4 -4 0 2 -1 0", "10", "7"], ["0 4 -4 0 4 -4 0 2 -1 0", "10", "7"], ["0 4 0 4 0 -2 2 0", "10", "7"], ["0 -3 4 0 4 0 -2 2 0", "10", "7"], ["0 4 -3 0 4 0 -2 2 0", "10", "7"], ["0 -4 4 0 4 0 -2 2 0", "10", "7"], ["0 4 -4 0 4 0 -2 2 0", "10", "7"], ["0 4 0 -3 4 0 -2 2 0", "10", "7"], ["0 -3 4 0 -3 4 0 -2 2 0", "10", "7"], ["0 4 -3 0 -3 4 0 -2 2 0", "10", "7"], ["0 -4 4 0 -3 4 0 -2 2 0", "10", "7"], ["0 4 -4 0 -3 4 0 -2 2 0", "10", "7"], ["0 4 0 4 -3 0 -2 2 0", "10", "7"], ["0 -3 4 0 4 -3 0 -2 2 0", "10", "7"], ["0 4 -3 0 4 -3 0 -2 2 0", "10", "7"], ["0 -4 4 0 4 -3 0 -2 2 0", "10", "7"], ["0 4 -4 0 4 -3 0 -2 2 0", "10", "7"], ["0 4 0 -4 4 0 -2 2 0", "10", "7"], ["0 -3 4 0 -4 4 0 -2 2 0", "10", "7"], ["0 4 -3 0 -4 4 0 -2 2 0", "10", "7"], ["0 -4 4 0 -4 4 0 -2 2 0", "10", "7"], ["0 4 -4 0 -4 4 0 -2 2 0", "10", "7"], ["0 4 0 4 -4 0 -2 2 0", "10", "7"], ["0 -3 4 0 4 -4 0 -2 2 0", "10", "7"], ["0 4 -3 0 4 -4 0 -2 2 0", "10", "7"], ["0 -4 4 0 4 -4 0 -2 2 0", "10", "7"], ["0 4 -4 0 4 -4 0 -2 2 0", "10", "7"], ["0 4 0 4 0 2 -2 0", "10", "7"], ["0 -3 4 0 4 0 2 -2 0", "10", "7"], ["0 4 -3 0 4 0 2 -2 0", "10", "7"], ["0 -4 4 0 4 0 2 -2 0", "10", "7"], ["0 4 -4 0 4 0 2 -2 0", "10", "7"], ["0 4 0 -3 4 0 2 -2 0", "10", "7"], ["0 -3 4 0 -3 4 0 2 -2 0", "10", "7"], ["0 4 -3 0 -3 4 0 2 -2 0", "10", "7"], ["0 -4 4 0 -3 4 0 2 -2 0", "10", "7"], ["0 4 -4 0 -3 4 0 2 -2 0", "10", "7"], ["0 4 0 4 -3 0 2 -2 0", "10", "7"], ["0 -3 4 0 4 -3 0 2 -2 0", "10", "7"], ["0 4 -3 0 4 -3 0 2 -2 0", "10", "7"], ["0 -4 4 0 4 -3 0 2 -2 0", "10", "7"], ["0 4 -4 0 4 -3 0 2 -2 0", "10", "7"], ["0 4 0 -4 4 0 2 -2 0", "10", "7"], ["0 -3 4 0 -4 4 0 2 -2 0", "10", "7"], ["0 4 -3 0 -4 4 0 2 -2 0", "10", "7"], ["0 -4 4 0 -4 4 0 2 -2 0", "10", "7"], ["0 4 -4 0 -4 4 0 2 -2 0", "10", "7"], ["0 4 0 4 -4 0 2 -2 0", "10", "7"], ["0 -3 4 0 4 -4 0 2 -2 0", "10", "7"], ["0 4 -3 0 4 -4 0 2 -2 0", "10", "7"], ["0 -4 4 0 4 -4 0 2 -2 0", "10", "7"], ["0 4 -4 0 4 -4 0 2 -2 0", "10", "7"], ["0 4 0 2 0 4 0", "10", "8"], ["0 -3 4 0 2 0 4 0", "10", "8"], ["0 4 -3 0 2 0 4 0", "10", "8"], ["0 -4 4 0 2 0 4 0", "10", "8"], ["0 4 -4 0 2 0 4 0", "10", "8"], ["0 4 0 -1 2 0 4 0", "10", "8"], ["0 -3 4 0 -1 2 0 4 0", "10", "8"], ["0 4 -3 0 -1 2 0 4 0", "10", "8"], ["0 -4 4 0 -1 2 0 4 0", "10", "8"], ["0 4 -4 0 -1 2 0 4 0", "10", "8"], ["0 4 0 2 -1 0 4 0", "10", "8"], ["0 -3 4 0 2 -1 0 4 0", "10", "8"], ["0 4 -3 0 2 -1 0 4 0", "10", "8"], ["0 -4 4 0 2 -1 0 4 0", "10", "8"], ["0 4 -4 0 2 -1 0 4 0", "10", "8"], ["0 4 0 -2 2 0 4 0", "10", "8"], ["0 -3 4 0 -2 2 0 4 0", "10", "8"], ["0 4 -3 0 -2 2 0 4 0", "10", "8"], ["0 -4 4 0 -2 2 0 4 0", "10", "8"], ["0 4 -4 0 -2 2 0 4 0", "10", "8"], ["0 4 0 2 -2 0 4 0", "10", "8"], ["0 -3 4 0 2 -2 0 4 0", "10", "8"], ["0 4 -3 0 2 -2 0 4 0", "10", "8"], ["0 -4 4 0 2 -2 0 4 0", "10", "8"], ["0 4 -4 0 2 -2 0 4 0", "10", "8"], ["0 4 0 2 0 -3 4 0", "10", "8"], ["0 -3 4 0 2 0 -3 4 0", "10", "8"], ["0 4 -3 0 2 0 -3 4 0", "10", "8"], ["0 -4 4 0 2 0 -3 4 0", "10", "8"], ["0 4 -4 0 2 0 -3 4 0", "10", "8"], ["0 4 0 -1 2 0 -3 4 0", "10", "8"], ["0 -3 4 0 -1 2 0 -3 4 0", "10", "8"], ["0 4 -3 0 -1 2 0 -3 4 0", "10", "8"], ["0 -4 4 0 -1 2 0 -3 4 0", "10", "8"], ["0 4 -4 0 -1 2 0 -3 4 0", "10", "8"], ["0 4 0 2 -1 0 -3 4 0", "10", "8"], ["0 -3 4 0 2 -1 0 -3 4 0", "10", "8"], ["0 4 -3 0 2 -1 0 -3 4 0", "10", "8"], ["0 -4 4 0 2 -1 0 -3 4 0", "10", "8"], ["0 4 -4 0 2 -1 0 -3 4 0", "10", "8"], ["0 4 0 -2 2 0 -3 4 0", "10", "8"], ["0 -3 4 0 -2 2 0 -3 4 0", "10", "8"], ["0 4 -3 0 -2 2 0 -3 4 0", "10", "8"], ["0 -4 4 0 -2 2 0 -3 4 0", "10", "8"], ["0 4 -4 0 -2 2 0 -3 4 0", "10", "8"], ["0 4 0 2 -2 0 -3 4 0", "10", "8"], ["0 -3 4 0 2 -2 0 -3 4 0", "10", "8"], ["0 4 -3 0 2 -2 0 -3 4 0", "10", "8"], ["0 -4 4 0 2 -2 0 -3 4 0", "10", "8"], ["0 4 -4 0 2 -2 0 -3 4 0", "10", "8"], ["0 4 0 2 0 4 -3 0", "10", "8"], ["0 -3 4 0 2 0 4 -3 0", "10", "8"], ["0 4 -3 0 2 0 4 -3 0", "10", "8"], ["0 -4 4 0 2 0 4 -3 0", "10", "8"], ["0 4 -4 0 2 0 4 -3 0", "10", "8"], ["0 4 0 -1 2 0 4 -3 0", "10", "8"], ["0 -3 4 0 -1 2 0 4 -3 0", "10", "8"], ["0 4 -3 0 -1 2 0 4 -3 0", "10", "8"], ["0 -4 4 0 -1 2 0 4 -3 0", "10", "8"], ["0 4 -4 0 -1 2 0 4 -3 0", "10", "8"], ["0 4 0 2 -1 0 4 -3 0", "10", "8"], ["0 -3 4 0 2 -1 0 4 -3 0", "10", "8"], ["0 4 -3 0 2 -1 0 4 -3 0", "10", "8"], ["0 -4 4 0 2 -1 0 4 -3 0", "10", "8"], ["0 4 -4 0 2 -1 0 4 -3 0", "10", "8"], ["0 4 0 -2 2 0 4 -3 0", "10", "8"], ["0 -3 4 0 -2 2 0 4 -3 0", "10", "8"], ["0 4 -3 0 -2 2 0 4 -3 0", "10", "8"], ["0 -4 4 0 -2 2 0 4 -3 0", "10", "8"], ["0 4 -4 0 -2 2 0 4 -3 0", "10", "8"], ["0 4 0 2 -2 0 4 -3 0", "10", "8"], ["0 -3 4 0 2 -2 0 4 -3 0", "10", "8"], ["0 4 -3 0 2 -2 0 4 -3 0", "10", "8"], ["0 -4 4 0 2 -2 0 4 -3 0", "10", "8"], ["0 4 -4 0 2 -2 0 4 -3 0", "10", "8"], ["0 4 0 2 0 -4 4 0", "10", "8"], ["0 -3 4 0 2 0 -4 4 0", "10", "8"], ["0 4 -3 0 2 0 -4 4 0", "10", "8"], ["0 -4 4 0 2 0 -4 4 0", "10", "8"], ["0 4 -4 0 2 0 -4 4 0", "10", "8"], ["0 4 0 -1 2 0 -4 4 0", "10", "8"], ["0 -3 4 0 -1 2 0 -4 4 0", "10", "8"], ["0 4 -3 0 -1 2 0 -4 4 0", "10", "8"], ["0 -4 4 0 -1 2 0 -4 4 0", "10", "8"], ["0 4 -4 0 -1 2 0 -4 4 0", "10", "8"], ["0 4 0 2 -1 0 -4 4 0", "10", "8"], ["0 -3 4 0 2 -1 0 -4 4 0", "10", "8"], ["0 4 -3 0 2 -1 0 -4 4 0", "10", "8"], ["0 -4 4 0 2 -1 0 -4 4 0", "10", "8"], ["0 4 -4 0 2 -1 0 -4 4 0", "10", "8"], ["0 4 0 -2 2 0 -4 4 0", "10", "8"], ["0 -3 4 0 -2 2 0 -4 4 0", "10", "8"], ["0 4 -3 0 -2 2 0 -4 4 0", "10", "8"], ["0 -4 4 0 -2 2 0 -4 4 0", "10", "8"], ["0 4 -4 0 -2 2 0 -4 4 0", "10", "8"], ["0 4 0 2 -2 0 -4 4 0", "10", "8"], ["0 -3 4 0 2 -2 0 -4 4 0", "10", "8"], ["0 4 -3 0 2 -2 0 -4 4 0", "10", "8"], ["0 -4 4 0 2 -2 0 -4 4 0", "10", "8"], ["0 4 -4 0 2 -2 0 -4 4 0", "10", "8"], ["0 4 0 2 0 4 -4 0", "10", "8"], ["0 -3 4 0 2 0 4 -4 0", "10", "8"], ["0 4 -3 0 2 0 4 -4 0", "10", "8"], ["0 -4 4 0 2 0 4 -4 0", "10", "8"], ["0 4 -4 0 2 0 4 -4 0", "10", "8"], ["0 4 0 -1 2 0 4 -4 0", "10", "8"], ["0 -3 4 0 -1 2 0 4 -4 0", "10", "8"], ["0 4 -3 0 -1 2 0 4 -4 0", "10", "8"], ["0 -4 4 0 -1 2 0 4 -4 0", "10", "8"], ["0 4 -4 0 -1 2 0 4 -4 0", "10", "8"], ["0 4 0 2 -1 0 4 -4 0", "10", "8"], ["0 -3 4 0 2 -1 0 4 -4 0", "10", "8"], ["0 4 -3 0 2 -1 0 4 -4 0", "10", "8"], ["0 -4 4 0 2 -1 0 4 -4 0", "10", "8"], ["0 4 -4 0 2 -1 0 4 -4 0", "10", "8"], ["0 4 0 -2 2 0 4 -4 0", "10", "8"], ["0 -3 4 0 -2 2 0 4 -4 0", "10", "8"], ["0 4 -3 0 -2 2 0 4 -4 0", "10", "8"], ["0 -4 4 0 -2 2 0 4 -4 0", "10", "8"], ["0 4 -4 0 -2 2 0 4 -4 0", "10", "8"], ["0 4 0 2 -2 0 4 -4 0", "10", "8"], ["0 -3 4 0 2 -2 0 4 -4 0", "10", "8"], ["0 4 -3 0 2 -2 0 4 -4 0", "10", "8"], ["0 -4 4 0 2 -2 0 4 -4 0", "10", "8"], ["0 4 -4 0 2 -2 0 4 -4 0", "10", "8"]]
  in  "4 groups":string[][](array[string])=[["0 1 0 1 0 3 0", "10", "1"], ["0 -1 1 0 1 0 3 0", "10", "1"], ["0 1 -1 0 1 0 3 0", "10", "1"], ["0 -4 1 0 1 0 3 0", "10", "1"], ["0 1 -4 0 1 0 3 0", "10", "1"], ["0 1 0 -1 1 0 3 0", "10", "1"], ["0 -1 1 0 -1 1 0 3 0", "10", "1"], ["0 1 -1 0 -1 1 0 3 0", "10", "1"], ["0 -4 1 0 -1 1 0 3 0", "10", "1"], ["0 1 -4 0 -1 1 0 3 0", "10", "1"], ["0 1 0 1 -1 0 3 0", "10", "1"], ["0 -1 1 0 1 -1 0 3 0", "10", "1"], ["0 1 -1 0 1 -1 0 3 0", "10", "1"], ["0 -4 1 0 1 -1 0 3 0", "10", "1"], ["0 1 -4 0 1 -1 0 3 0", "10", "1"], ["0 1 0 -4 1 0 3 0", "10", "1"], ["0 -1 1 0 -4 1 0 3 0", "10", "1"], ["0 1 -1 0 -4 1 0 3 0", "10", "1"], ["0 -4 1 0 -4 1 0 3 0", "10", "1"], ["0 1 -4 0 -4 1 0 3 0", "10", "1"], ["0 1 0 1 -4 0 3 0", "10", "1"], ["0 -1 1 0 1 -4 0 3 0", "10", "1"], ["0 1 -1 0 1 -4 0 3 0", "10", "1"], ["0 -4 1 0 1 -4 0 3 0", "10", "1"], ["0 1 -4 0 1 -4 0 3 0", "10", "1"], ["0 1 0 1 0 -2 3 0", "10", "1"], ["0 -1 1 0 1 0 -2 3 0", "10", "1"], ["0 1 -1 0 1 0 -2 3 0", "10", "1"], ["0 -4 1 0 1 0 -2 3 0", "10", "1"], ["0 1 -4 0 1 0 -2 3 0", "10", "1"], ["0 1 0 -1 1 0 -2 3 0", "10", "1"], ["0 -1 1 0 -1 1 0 -2 3 0", "10", "1"], ["0 1 -1 0 -1 1 0 -2 3 0", "10", "1"], ["0 -4 1 0 -1 1 0 -2 3 0", "10", "1"], ["0 1 -4 0 -1 1 0 -2 3 0", "10", "1"], ["0 1 0 1 -1 0 -2 3 0", "10", "1"], ["0 -1 1 0 1 -1 0 -2 3 0", "10", "1"], ["0 1 -1 0 1 -1 0 -2 3 0", "10", "1"], ["0 -4 1 0 1 -1 0 -2 3 0", "10", "1"], ["0 1 -4 0 1 -1 0 -2 3 0", "10", "1"], ["0 1 0 -4 1 0 -2 3 0", "10", "1"], ["0 -1 1 0 -4 1 0 -2 3 0", "10", "1"], ["0 1 -1 0 -4 1 0 -2 3 0", "10", "1"], ["0 -4 1 0 -4 1 0 -2 3 0", "10", "1"], ["0 1 -4 0 -4 1 0 -2 3 0", "10", "1"], ["0 1 0 1 -4 0 -2 3 0", "10", "1"], ["0 -1 1 0 1 -4 0 -2 3 0", "10", "1"], ["0 1 -1 0 1 -4 0 -2 3 0", "10", "1"], ["0 -4 1 0 1 -4 0 -2 3 0", "10", "1"], ["0 1 -4 0 1 -4 0 -2 3 0", "10", "1"], ["0 1 0 1 0 3 -2 0", "10", "1"], ["0 -1 1 0 1 0 3 -2 0", "10", "1"], ["0 1 -1 0 1 0 3 -2 0", "10", "1"], ["0 -4 1 0 1 0 3 -2 0", "10", "1"], ["0 1 -4 0 1 0 3 -2 0", "10", "1"], ["0 1 0 -1 1 0 3 -2 0", "10", "1"], ["0 -1 1 0 -1 1 0 3 -2 0", "10", "1"], ["0 1 -1 0 -1 1 0 3 -2 0", "10", "1"], ["0 -4 1 0 -1 1 0 3 -2 0", "10", "1"], ["0 1 -4 0 -1 1 0 3 -2 0", "10", "1"], ["0 1 0 1 -1 0 3 -2 0", "10", "1"], ["0 -1 1 0 1 -1 0 3 -2 0", "10", "1"], ["0 1 -1 0 1 -1 0 3 -2 0", "10", "1"], ["0 -4 1 0 1 -1 0 3 -2 0", "10", "1"], ["0 1 -4 0 1 -1 0 3 -2 0", "10", "1"], ["0 1 0 -4 1 0 3 -2 0", "10", "1"], ["0 -1 1 0 -4 1 0 3 -2 0", "10", "1"], ["0 1 -1 0 -4 1 0 3 -2 0", "10", "1"], ["0 -4 1 0 -4 1 0 3 -2 0", "10", "1"], ["0 1 -4 0 -4 1 0 3 -2 0", "10", "1"], ["0 1 0 1 -4 0 3 -2 0", "10", "1"], ["0 -1 1 0 1 -4 0 3 -2 0", "10", "1"], ["0 1 -1 0 1 -4 0 3 -2 0", "10", "1"], ["0 -4 1 0 1 -4 0 3 -2 0", "10", "1"], ["0 1 -4 0 1 -4 0 3 -2 0", "10", "1"], ["0 1 0 1 0 -3 3 0", "10", "1"], ["0 -1 1 0 1 0 -3 3 0", "10", "1"], ["0 1 -1 0 1 0 -3 3 0", "10", "1"], ["0 -4 1 0 1 0 -3 3 0", "10", "1"], ["0 1 -4 0 1 0 -3 3 0", "10", "1"], ["0 1 0 -1 1 0 -3 3 0", "10", "1"], ["0 -1 1 0 -1 1 0 -3 3 0", "10", "1"], ["0 1 -1 0 -1 1 0 -3 3 0", "10", "1"], ["0 -4 1 0 -1 1 0 -3 3 0", "10", "1"], ["0 1 -4 0 -1 1 0 -3 3 0", "10", "1"], ["0 1 0 1 -1 0 -3 3 0", "10", "1"], ["0 -1 1 0 1 -1 0 -3 3 0", "10", "1"], ["0 1 -1 0 1 -1 0 -3 3 0", "10", "1"], ["0 -4 1 0 1 -1 0 -3 3 0", "10", "1"], ["0 1 -4 0 1 -1 0 -3 3 0", "10", "1"], ["0 1 0 -4 1 0 -3 3 0", "10", "1"], ["0 -1 1 0 -4 1 0 -3 3 0", "10", "1"], ["0 1 -1 0 -4 1 0 -3 3 0", "10", "1"], ["0 -4 1 0 -4 1 0 -3 3 0", "10", "1"], ["0 1 -4 0 -4 1 0 -3 3 0", "10", "1"], ["0 1 0 1 -4 0 -3 3 0", "10", "1"], ["0 -1 1 0 1 -4 0 -3 3 0", "10", "1"], ["0 1 -1 0 1 -4 0 -3 3 0", "10", "1"], ["0 -4 1 0 1 -4 0 -3 3 0", "10", "1"], ["0 1 -4 0 1 -4 0 -3 3 0", "10", "1"], ["0 1 0 1 0 3 -3 0", "10", "1"], ["0 -1 1 0 1 0 3 -3 0", "10", "1"], ["0 1 -1 0 1 0 3 -3 0", "10", "1"], ["0 -4 1 0 1 0 3 -3 0", "10", "1"], ["0 1 -4 0 1 0 3 -3 0", "10", "1"], ["0 1 0 -1 1 0 3 -3 0", "10", "1"], ["0 -1 1 0 -1 1 0 3 -3 0", "10", "1"], ["0 1 -1 0 -1 1 0 3 -3 0", "10", "1"], ["0 -4 1 0 -1 1 0 3 -3 0", "10", "1"], ["0 1 -4 0 -1 1 0 3 -3 0", "10", "1"], ["0 1 0 1 -1 0 3 -3 0", "10", "1"], ["0 -1 1 0 1 -1 0 3 -3 0", "10", "1"], ["0 1 -1 0 1 -1 0 3 -3 0", "10", "1"], ["0 -4 1 0 1 -1 0 3 -3 0", "10", "1"], ["0 1 -4 0 1 -1 0 3 -3 0", "10", "1"], ["0 1 0 -4 1 0 3 -3 0", "10", "1"], ["0 -1 1 0 -4 1 0 3 -3 0", "10", "1"], ["0 1 -1 0 -4 1 0 3 -3 0", "10", "1"], ["0 -4 1 0 -4 1 0 3 -3 0", "10", "1"], ["0 1 -4 0 -4 1 0 3 -3 0", "10", "1"], ["0 1 0 1 -4 0 3 -3 0", "10", "1"], ["0 -1 1 0 1 -4 0 3 -3 0", "10", "1"], ["0 1 -1 0 1 -4 0 3 -3 0", "10", "1"], ["0 -4 1 0 1 -4 0 3 -3 0", "10", "1"], ["0 1 -4 0 1 -4 0 3 -3 0", "10", "1"], ["0 1 0 3 0 1 0", "10", "2"], ["0 -1 1 0 3 0 1 0", "10", "2"], ["0 1 -1 0 3 0 1 0", "10", "2"], ["0 -4 1 0 3 0 1 0", "10", "2"], ["0 1 -4 0 3 0 1 0", "10", "2"], ["0 1 0 -2 3 0 1 0", "10", "2"], ["0 -1 1 0 -2 3 0 1 0", "10", "2"], ["0 1 -1 0 -2 3 0 1 0", "10", "2"], ["0 -4 1 0 -2 3 0 1 0", "10", "2"], ["0 1 -4 0 -2 3 0 1 0", "10", "2"], ["0 1 0 3 -2 0 1 0", "10", "2"], ["0 -1 1 0 3 -2 0 1 0", "10", "2"], ["0 1 -1 0 3 -2 0 1 0", "10", "2"], ["0 -4 1 0 3 -2 0 1 0", "10", "2"], ["0 1 -4 0 3 -2 0 1 0", "10", "2"], ["0 1 0 -3 3 0 1 0", "10", "2"], ["0 -1 1 0 -3 3 0 1 0", "10", "2"], ["0 1 -1 0 -3 3 0 1 0", "10", "2"], ["0 -4 1 0 -3 3 0 1 0", "10", "2"], ["0 1 -4 0 -3 3 0 1 0", "10", "2"], ["0 1 0 3 -3 0 1 0", "10", "2"], ["0 -1 1 0 3 -3 0 1 0", "10", "2"], ["0 1 -1 0 3 -3 0 1 0", "10", "2"], ["0 -4 1 0 3 -3 0 1 0", "10", "2"], ["0 1 -4 0 3 -3 0 1 0", "10", "2"], ["0 1 0 3 0 -1 1 0", "10", "2"], ["0 -1 1 0 3 0 -1 1 0", "10", "2"], ["0 1 -1 0 3 0 -1 1 0", "10", "2"], ["0 -4 1 0 3 0 -1 1 0", "10", "2"], ["0 1 -4 0 3 0 -1 1 0", "10", "2"], ["0 1 0 -2 3 0 -1 1 0", "10", "2"], ["0 -1 1 0 -2 3 0 -1 1 0", "10", "2"], ["0 1 -1 0 -2 3 0 -1 1 0", "10", "2"], ["0 -4 1 0 -2 3 0 -1 1 0", "10", "2"], ["0 1 -4 0 -2 3 0 -1 1 0", "10", "2"], ["0 1 0 3 -2 0 -1 1 0", "10", "2"], ["0 -1 1 0 3 -2 0 -1 1 0", "10", "2"], ["0 1 -1 0 3 -2 0 -1 1 0", "10", "2"], ["0 -4 1 0 3 -2 0 -1 1 0", "10", "2"], ["0 1 -4 0 3 -2 0 -1 1 0", "10", "2"], ["0 1 0 -3 3 0 -1 1 0", "10", "2"], ["0 -1 1 0 -3 3 0 -1 1 0", "10", "2"], ["0 1 -1 0 -3 3 0 -1 1 0", "10", "2"], ["0 -4 1 0 -3 3 0 -1 1 0", "10", "2"], ["0 1 -4 0 -3 3 0 -1 1 0", "10", "2"], ["0 1 0 3 -3 0 -1 1 0", "10", "2"], ["0 -1 1 0 3 -3 0 -1 1 0", "10", "2"], ["0 1 -1 0 3 -3 0 -1 1 0", "10", "2"], ["0 -4 1 0 3 -3 0 -1 1 0", "10", "2"], ["0 1 -4 0 3 -3 0 -1 1 0", "10", "2"], ["0 1 0 3 0 1 -1 0", "10", "2"], ["0 -1 1 0 3 0 1 -1 0", "10", "2"], ["0 1 -1 0 3 0 1 -1 0", "10", "2"], ["0 -4 1 0 3 0 1 -1 0", "10", "2"], ["0 1 -4 0 3 0 1 -1 0", "10", "2"], ["0 1 0 -2 3 0 1 -1 0", "10", "2"], ["0 -1 1 0 -2 3 0 1 -1 0", "10", "2"], ["0 1 -1 0 -2 3 0 1 -1 0", "10", "2"], ["0 -4 1 0 -2 3 0 1 -1 0", "10", "2"], ["0 1 -4 0 -2 3 0 1 -1 0", "10", "2"], ["0 1 0 3 -2 0 1 -1 0", "10", "2"], ["0 -1 1 0 3 -2 0 1 -1 0", "10", "2"], ["0 1 -1 0 3 -2 0 1 -1 0", "10", "2"], ["0 -4 1 0 3 -2 0 1 -1 0", "10", "2"], ["0 1 -4 0 3 -2 0 1 -1 0", "10", "2"], ["0 1 0 -3 3 0 1 -1 0", "10", "2"], ["0 -1 1 0 -3 3 0 1 -1 0", "10", "2"], ["0 1 -1 0 -3 3 0 1 -1 0", "10", "2"], ["0 -4 1 0 -3 3 0 1 -1 0", "10", "2"], ["0 1 -4 0 -3 3 0 1 -1 0", "10", "2"], ["0 1 0 3 -3 0 1 -1 0", "10", "2"], ["0 -1 1 0 3 -3 0 1 -1 0", "10", "2"], ["0 1 -1 0 3 -3 0 1 -1 0", "10", "2"], ["0 -4 1 0 3 -3 0 1 -1 0", "10", "2"], ["0 1 -4 0 3 -3 0 1 -1 0", "10", "2"], ["0 1 0 3 0 -4 1 0", "10", "2"], ["0 -1 1 0 3 0 -4 1 0", "10", "2"], ["0 1 -1 0 3 0 -4 1 0", "10", "2"], ["0 -4 1 0 3 0 -4 1 0", "10", "2"], ["0 1 -4 0 3 0 -4 1 0", "10", "2"], ["0 1 0 -2 3 0 -4 1 0", "10", "2"], ["0 -1 1 0 -2 3 0 -4 1 0", "10", "2"], ["0 1 -1 0 -2 3 0 -4 1 0", "10", "2"], ["0 -4 1 0 -2 3 0 -4 1 0", "10", "2"], ["0 1 -4 0 -2 3 0 -4 1 0", "10", "2"], ["0 1 0 3 -2 0 -4 1 0", "10", "2"], ["0 -1 1 0 3 -2 0 -4 1 0", "10", "2"], ["0 1 -1 0 3 -2 0 -4 1 0", "10", "2"], ["0 -4 1 0 3 -2 0 -4 1 0", "10", "2"], ["0 1 -4 0 3 -2 0 -4 1 0", "10", "2"], ["0 1 0 -3 3 0 -4 1 0", "10", "2"], ["0 -1 1 0 -3 3 0 -4 1 0", "10", "2"], ["0 1 -1 0 -3 3 0 -4 1 0", "10", "2"], ["0 -4 1 0 -3 3 0 -4 1 0", "10", "2"], ["0 1 -4 0 -3 3 0 -4 1 0", "10", "2"], ["0 1 0 3 -3 0 -4 1 0", "10", "2"], ["0 -1 1 0 3 -3 0 -4 1 0", "10", "2"], ["0 1 -1 0 3 -3 0 -4 1 0", "10", "2"], ["0 -4 1 0 3 -3 0 -4 1 0", "10", "2"], ["0 1 -4 0 3 -3 0 -4 1 0", "10", "2"], ["0 1 0 3 0 1 -4 0", "10", "2"], ["0 -1 1 0 3 0 1 -4 0", "10", "2"], ["0 1 -1 0 3 0 1 -4 0", "10", "2"], ["0 -4 1 0 3 0 1 -4 0", "10", "2"], ["0 1 -4 0 3 0 1 -4 0", "10", "2"], ["0 1 0 -2 3 0 1 -4 0", "10", "2"], ["0 -1 1 0 -2 3 0 1 -4 0", "10", "2"], ["0 1 -1 0 -2 3 0 1 -4 0", "10", "2"], ["0 -4 1 0 -2 3 0 1 -4 0", "10", "2"], ["0 1 -4 0 -2 3 0 1 -4 0", "10", "2"], ["0 1 0 3 -2 0 1 -4 0", "10", "2"], ["0 -1 1 0 3 -2 0 1 -4 0", "10", "2"], ["0 1 -1 0 3 -2 0 1 -4 0", "10", "2"], ["0 -4 1 0 3 -2 0 1 -4 0", "10", "2"], ["0 1 -4 0 3 -2 0 1 -4 0", "10", "2"], ["0 1 0 -3 3 0 1 -4 0", "10", "2"], ["0 -1 1 0 -3 3 0 1 -4 0", "10", "2"], ["0 1 -1 0 -3 3 0 1 -4 0", "10", "2"], ["0 -4 1 0 -3 3 0 1 -4 0", "10", "2"], ["0 1 -4 0 -3 3 0 1 -4 0", "10", "2"], ["0 1 0 3 -3 0 1 -4 0", "10", "2"], ["0 -1 1 0 3 -3 0 1 -4 0", "10", "2"], ["0 1 -1 0 3 -3 0 1 -4 0", "10", "2"], ["0 -4 1 0 3 -3 0 1 -4 0", "10", "2"], ["0 1 -4 0 3 -3 0 1 -4 0", "10", "2"], ["0 3 0 3 0 1 0", "10", "3"], ["0 -2 3 0 3 0 1 0", "10", "3"], ["0 3 -2 0 3 0 1 0", "10", "3"], ["0 -3 3 0 3 0 1 0", "10", "3"], ["0 3-3 0 3 0 1 0", "10", "3"], ["0 3 0 -2 3 0 1 0", "10", "3"], ["0 -2 3 0 -2 3 0 1 0", "10", "3"], ["0 3 -2 0 -2 3 0 1 0", "10", "3"], ["0 -3 3 0 -2 3 0 1 0", "10", "3"], ["0 3-3 0 -2 3 0 1 0", "10", "3"], ["0 3 0 3 -2 0 1 0", "10", "3"], ["0 -2 3 0 3 -2 0 1 0", "10", "3"], ["0 3 -2 0 3 -2 0 1 0", "10", "3"], ["0 -3 3 0 3 -2 0 1 0", "10", "3"], ["0 3-3 0 3 -2 0 1 0", "10", "3"], ["0 3 0 -3 3 0 1 0", "10", "3"], ["0 -2 3 0 -3 3 0 1 0", "10", "3"], ["0 3 -2 0 -3 3 0 1 0", "10", "3"], ["0 -3 3 0 -3 3 0 1 0", "10", "3"], ["0 3-3 0 -3 3 0 1 0", "10", "3"], ["0 3 0 3 -3 0 1 0", "10", "3"], ["0 -2 3 0 3 -3 0 1 0", "10", "3"], ["0 3 -2 0 3 -3 0 1 0", "10", "3"], ["0 -3 3 0 3 -3 0 1 0", "10", "3"], ["0 3-3 0 3 -3 0 1 0", "10", "3"], ["0 3 0 3 0 -1 1 0", "10", "3"], ["0 -2 3 0 3 0 -1 1 0", "10", "3"], ["0 3 -2 0 3 0 -1 1 0", "10", "3"], ["0 -3 3 0 3 0 -1 1 0", "10", "3"], ["0 3-3 0 3 0 -1 1 0", "10", "3"], ["0 3 0 -2 3 0 -1 1 0", "10", "3"], ["0 -2 3 0 -2 3 0 -1 1 0", "10", "3"], ["0 3 -2 0 -2 3 0 -1 1 0", "10", "3"], ["0 -3 3 0 -2 3 0 -1 1 0", "10", "3"], ["0 3-3 0 -2 3 0 -1 1 0", "10", "3"], ["0 3 0 3 -2 0 -1 1 0", "10", "3"], ["0 -2 3 0 3 -2 0 -1 1 0", "10", "3"], ["0 3 -2 0 3 -2 0 -1 1 0", "10", "3"], ["0 -3 3 0 3 -2 0 -1 1 0", "10", "3"], ["0 3-3 0 3 -2 0 -1 1 0", "10", "3"], ["0 3 0 -3 3 0 -1 1 0", "10", "3"], ["0 -2 3 0 -3 3 0 -1 1 0", "10", "3"], ["0 3 -2 0 -3 3 0 -1 1 0", "10", "3"], ["0 -3 3 0 -3 3 0 -1 1 0", "10", "3"], ["0 3-3 0 -3 3 0 -1 1 0", "10", "3"], ["0 3 0 3 -3 0 -1 1 0", "10", "3"], ["0 -2 3 0 3 -3 0 -1 1 0", "10", "3"], ["0 3 -2 0 3 -3 0 -1 1 0", "10", "3"], ["0 -3 3 0 3 -3 0 -1 1 0", "10", "3"], ["0 3-3 0 3 -3 0 -1 1 0", "10", "3"], ["0 3 0 3 0 1 -1 0", "10", "3"], ["0 -2 3 0 3 0 1 -1 0", "10", "3"], ["0 3 -2 0 3 0 1 -1 0", "10", "3"], ["0 -3 3 0 3 0 1 -1 0", "10", "3"], ["0 3-3 0 3 0 1 -1 0", "10", "3"], ["0 3 0 -2 3 0 1 -1 0", "10", "3"], ["0 -2 3 0 -2 3 0 1 -1 0", "10", "3"], ["0 3 -2 0 -2 3 0 1 -1 0", "10", "3"], ["0 -3 3 0 -2 3 0 1 -1 0", "10", "3"], ["0 3-3 0 -2 3 0 1 -1 0", "10", "3"], ["0 3 0 3 -2 0 1 -1 0", "10", "3"], ["0 -2 3 0 3 -2 0 1 -1 0", "10", "3"], ["0 3 -2 0 3 -2 0 1 -1 0", "10", "3"], ["0 -3 3 0 3 -2 0 1 -1 0", "10", "3"], ["0 3-3 0 3 -2 0 1 -1 0", "10", "3"], ["0 3 0 -3 3 0 1 -1 0", "10", "3"], ["0 -2 3 0 -3 3 0 1 -1 0", "10", "3"], ["0 3 -2 0 -3 3 0 1 -1 0", "10", "3"], ["0 -3 3 0 -3 3 0 1 -1 0", "10", "3"], ["0 3-3 0 -3 3 0 1 -1 0", "10", "3"], ["0 3 0 3 -3 0 1 -1 0", "10", "3"], ["0 -2 3 0 3 -3 0 1 -1 0", "10", "3"], ["0 3 -2 0 3 -3 0 1 -1 0", "10", "3"], ["0 -3 3 0 3 -3 0 1 -1 0", "10", "3"], ["0 3-3 0 3 -3 0 1 -1 0", "10", "3"], ["0 3 0 3 0 -4 1 0", "10", "3"], ["0 -2 3 0 3 0 -4 1 0", "10", "3"], ["0 3 -2 0 3 0 -4 1 0", "10", "3"], ["0 -3 3 0 3 0 -4 1 0", "10", "3"], ["0 3-3 0 3 0 -4 1 0", "10", "3"], ["0 3 0 -2 3 0 -4 1 0", "10", "3"], ["0 -2 3 0 -2 3 0 -4 1 0", "10", "3"], ["0 3 -2 0 -2 3 0 -4 1 0", "10", "3"], ["0 -3 3 0 -2 3 0 -4 1 0", "10", "3"], ["0 3-3 0 -2 3 0 -4 1 0", "10", "3"], ["0 3 0 3 -2 0 -4 1 0", "10", "3"], ["0 -2 3 0 3 -2 0 -4 1 0", "10", "3"], ["0 3 -2 0 3 -2 0 -4 1 0", "10", "3"], ["0 -3 3 0 3 -2 0 -4 1 0", "10", "3"], ["0 3-3 0 3 -2 0 -4 1 0", "10", "3"], ["0 3 0 -3 3 0 -4 1 0", "10", "3"], ["0 -2 3 0 -3 3 0 -4 1 0", "10", "3"], ["0 3 -2 0 -3 3 0 -4 1 0", "10", "3"], ["0 -3 3 0 -3 3 0 -4 1 0", "10", "3"], ["0 3-3 0 -3 3 0 -4 1 0", "10", "3"], ["0 3 0 3 -3 0 -4 1 0", "10", "3"], ["0 -2 3 0 3 -3 0 -4 1 0", "10", "3"], ["0 3 -2 0 3 -3 0 -4 1 0", "10", "3"], ["0 -3 3 0 3 -3 0 -4 1 0", "10", "3"], ["0 3-3 0 3 -3 0 -4 1 0", "10", "3"], ["0 3 0 3 0 1 -4 0", "10", "3"], ["0 -2 3 0 3 0 1 -4 0", "10", "3"], ["0 3 -2 0 3 0 1 -4 0", "10", "3"], ["0 -3 3 0 3 0 1 -4 0", "10", "3"], ["0 3-3 0 3 0 1 -4 0", "10", "3"], ["0 3 0 -2 3 0 1 -4 0", "10", "3"], ["0 -2 3 0 -2 3 0 1 -4 0", "10", "3"], ["0 3 -2 0 -2 3 0 1 -4 0", "10", "3"], ["0 -3 3 0 -2 3 0 1 -4 0", "10", "3"], ["0 3-3 0 -2 3 0 1 -4 0", "10", "3"], ["0 3 0 3 -2 0 1 -4 0", "10", "3"], ["0 -2 3 0 3 -2 0 1 -4 0", "10", "3"], ["0 3 -2 0 3 -2 0 1 -4 0", "10", "3"], ["0 -3 3 0 3 -2 0 1 -4 0", "10", "3"], ["0 3-3 0 3 -2 0 1 -4 0", "10", "3"], ["0 3 0 -3 3 0 1 -4 0", "10", "3"], ["0 -2 3 0 -3 3 0 1 -4 0", "10", "3"], ["0 3 -2 0 -3 3 0 1 -4 0", "10", "3"], ["0 -3 3 0 -3 3 0 1 -4 0", "10", "3"], ["0 3-3 0 -3 3 0 1 -4 0", "10", "3"], ["0 3 0 3 -3 0 1 -4 0", "10", "3"], ["0 -2 3 0 3 -3 0 1 -4 0", "10", "3"], ["0 3 -2 0 3 -3 0 1 -4 0", "10", "3"], ["0 -3 3 0 3 -3 0 1 -4 0", "10", "3"], ["0 3-3 0 3 -3 0 1 -4 0", "10", "3"], ["0 3 0 1 0 3 0", "10", "4"], ["0 -2 3 0 1 0 3 0", "10", "4"], ["0 3 -2 0 1 0 3 0", "10", "4"], ["0 -3 3 0 1 0 3 0", "10", "4"], ["0 3-3 0 1 0 3 0", "10", "4"], ["0 3 0 -1 1 0 3 0", "10", "4"], ["0 -2 3 0 -1 1 0 3 0", "10", "4"], ["0 3 -2 0 -1 1 0 3 0", "10", "4"], ["0 -3 3 0 -1 1 0 3 0", "10", "4"], ["0 3-3 0 -1 1 0 3 0", "10", "4"], ["0 3 0 1 -1 0 3 0", "10", "4"], ["0 -2 3 0 1 -1 0 3 0", "10", "4"], ["0 3 -2 0 1 -1 0 3 0", "10", "4"], ["0 -3 3 0 1 -1 0 3 0", "10", "4"], ["0 3-3 0 1 -1 0 3 0", "10", "4"], ["0 3 0 -4 1 0 3 0", "10", "4"], ["0 -2 3 0 -4 1 0 3 0", "10", "4"], ["0 3 -2 0 -4 1 0 3 0", "10", "4"], ["0 -3 3 0 -4 1 0 3 0", "10", "4"], ["0 3-3 0 -4 1 0 3 0", "10", "4"], ["0 3 0 1 -4 0 3 0", "10", "4"], ["0 -2 3 0 1 -4 0 3 0", "10", "4"], ["0 3 -2 0 1 -4 0 3 0", "10", "4"], ["0 -3 3 0 1 -4 0 3 0", "10", "4"], ["0 3-3 0 1 -4 0 3 0", "10", "4"], ["0 3 0 1 0 -2 3 0", "10", "4"], ["0 -2 3 0 1 0 -2 3 0", "10", "4"], ["0 3 -2 0 1 0 -2 3 0", "10", "4"], ["0 -3 3 0 1 0 -2 3 0", "10", "4"], ["0 3-3 0 1 0 -2 3 0", "10", "4"], ["0 3 0 -1 1 0 -2 3 0", "10", "4"], ["0 -2 3 0 -1 1 0 -2 3 0", "10", "4"], ["0 3 -2 0 -1 1 0 -2 3 0", "10", "4"], ["0 -3 3 0 -1 1 0 -2 3 0", "10", "4"], ["0 3-3 0 -1 1 0 -2 3 0", "10", "4"], ["0 3 0 1 -1 0 -2 3 0", "10", "4"], ["0 -2 3 0 1 -1 0 -2 3 0", "10", "4"], ["0 3 -2 0 1 -1 0 -2 3 0", "10", "4"], ["0 -3 3 0 1 -1 0 -2 3 0", "10", "4"], ["0 3-3 0 1 -1 0 -2 3 0", "10", "4"], ["0 3 0 -4 1 0 -2 3 0", "10", "4"], ["0 -2 3 0 -4 1 0 -2 3 0", "10", "4"], ["0 3 -2 0 -4 1 0 -2 3 0", "10", "4"], ["0 -3 3 0 -4 1 0 -2 3 0", "10", "4"], ["0 3-3 0 -4 1 0 -2 3 0", "10", "4"], ["0 3 0 1 -4 0 -2 3 0", "10", "4"], ["0 -2 3 0 1 -4 0 -2 3 0", "10", "4"], ["0 3 -2 0 1 -4 0 -2 3 0", "10", "4"], ["0 -3 3 0 1 -4 0 -2 3 0", "10", "4"], ["0 3-3 0 1 -4 0 -2 3 0", "10", "4"], ["0 3 0 1 0 3 -2 0", "10", "4"], ["0 -2 3 0 1 0 3 -2 0", "10", "4"], ["0 3 -2 0 1 0 3 -2 0", "10", "4"], ["0 -3 3 0 1 0 3 -2 0", "10", "4"], ["0 3-3 0 1 0 3 -2 0", "10", "4"], ["0 3 0 -1 1 0 3 -2 0", "10", "4"], ["0 -2 3 0 -1 1 0 3 -2 0", "10", "4"], ["0 3 -2 0 -1 1 0 3 -2 0", "10", "4"], ["0 -3 3 0 -1 1 0 3 -2 0", "10", "4"], ["0 3-3 0 -1 1 0 3 -2 0", "10", "4"], ["0 3 0 1 -1 0 3 -2 0", "10", "4"], ["0 -2 3 0 1 -1 0 3 -2 0", "10", "4"], ["0 3 -2 0 1 -1 0 3 -2 0", "10", "4"], ["0 -3 3 0 1 -1 0 3 -2 0", "10", "4"], ["0 3-3 0 1 -1 0 3 -2 0", "10", "4"], ["0 3 0 -4 1 0 3 -2 0", "10", "4"], ["0 -2 3 0 -4 1 0 3 -2 0", "10", "4"], ["0 3 -2 0 -4 1 0 3 -2 0", "10", "4"], ["0 -3 3 0 -4 1 0 3 -2 0", "10", "4"], ["0 3-3 0 -4 1 0 3 -2 0", "10", "4"], ["0 3 0 1 -4 0 3 -2 0", "10", "4"], ["0 -2 3 0 1 -4 0 3 -2 0", "10", "4"], ["0 3 -2 0 1 -4 0 3 -2 0", "10", "4"], ["0 -3 3 0 1 -4 0 3 -2 0", "10", "4"], ["0 3-3 0 1 -4 0 3 -2 0", "10", "4"], ["0 3 0 1 0 -3 3 0", "10", "4"], ["0 -2 3 0 1 0 -3 3 0", "10", "4"], ["0 3 -2 0 1 0 -3 3 0", "10", "4"], ["0 -3 3 0 1 0 -3 3 0", "10", "4"], ["0 3-3 0 1 0 -3 3 0", "10", "4"], ["0 3 0 -1 1 0 -3 3 0", "10", "4"], ["0 -2 3 0 -1 1 0 -3 3 0", "10", "4"], ["0 3 -2 0 -1 1 0 -3 3 0", "10", "4"], ["0 -3 3 0 -1 1 0 -3 3 0", "10", "4"], ["0 3-3 0 -1 1 0 -3 3 0", "10", "4"], ["0 3 0 1 -1 0 -3 3 0", "10", "4"], ["0 -2 3 0 1 -1 0 -3 3 0", "10", "4"], ["0 3 -2 0 1 -1 0 -3 3 0", "10", "4"], ["0 -3 3 0 1 -1 0 -3 3 0", "10", "4"], ["0 3-3 0 1 -1 0 -3 3 0", "10", "4"], ["0 3 0 -4 1 0 -3 3 0", "10", "4"], ["0 -2 3 0 -4 1 0 -3 3 0", "10", "4"], ["0 3 -2 0 -4 1 0 -3 3 0", "10", "4"], ["0 -3 3 0 -4 1 0 -3 3 0", "10", "4"], ["0 3-3 0 -4 1 0 -3 3 0", "10", "4"], ["0 3 0 1 -4 0 -3 3 0", "10", "4"], ["0 -2 3 0 1 -4 0 -3 3 0", "10", "4"], ["0 3 -2 0 1 -4 0 -3 3 0", "10", "4"], ["0 -3 3 0 1 -4 0 -3 3 0", "10", "4"], ["0 3-3 0 1 -4 0 -3 3 0", "10", "4"], ["0 3 0 1 0 3 -3 0", "10", "4"], ["0 -2 3 0 1 0 3 -3 0", "10", "4"], ["0 3 -2 0 1 0 3 -3 0", "10", "4"], ["0 -3 3 0 1 0 3 -3 0", "10", "4"], ["0 3-3 0 1 0 3 -3 0", "10", "4"], ["0 3 0 -1 1 0 3 -3 0", "10", "4"], ["0 -2 3 0 -1 1 0 3 -3 0", "10", "4"], ["0 3 -2 0 -1 1 0 3 -3 0", "10", "4"], ["0 -3 3 0 -1 1 0 3 -3 0", "10", "4"], ["0 3-3 0 -1 1 0 3 -3 0", "10", "4"], ["0 3 0 1 -1 0 3 -3 0", "10", "4"], ["0 -2 3 0 1 -1 0 3 -3 0", "10", "4"], ["0 3 -2 0 1 -1 0 3 -3 0", "10", "4"], ["0 -3 3 0 1 -1 0 3 -3 0", "10", "4"], ["0 3-3 0 1 -1 0 3 -3 0", "10", "4"], ["0 3 0 -4 1 0 3 -3 0", "10", "4"], ["0 -2 3 0 -4 1 0 3 -3 0", "10", "4"], ["0 3 -2 0 -4 1 0 3 -3 0", "10", "4"], ["0 -3 3 0 -4 1 0 3 -3 0", "10", "4"], ["0 3-3 0 -4 1 0 3 -3 0", "10", "4"], ["0 3 0 1 -4 0 3 -3 0", "10", "4"], ["0 -2 3 0 1 -4 0 3 -3 0", "10", "4"], ["0 3 -2 0 1 -4 0 3 -3 0", "10", "4"], ["0 -3 3 0 1 -4 0 3 -3 0", "10", "4"], ["0 3-3 0 1 -4 0 3 -3 0", "10", "4"]]
  in  "cluster centers for dataset test":string[](array[string])=["0 -1 1 -4 0 -4 1 -1 0 -1 1 -4 0 -4 1 -1 0 -2 3 -3 0 -3 3 -2 0", "0 -1 1 -4 0 -4 1 -1 0 -2 3 -3 0 -3 3 -2 0 -1 1 -4 0 -4 1 -1 0", "0 -2 3 -3 0 -3 3 -2 0 -2 3 -3 0 -3 3 -2 0 -1 1 -4 0 -4 1 -1 0", "0 -2 3 -3 0 -3 3 -2 0 -1 1 -4 0 -4 1 -1 0 -2 3 -3 0 -3 3 -2 0", "0 -1 2 -2 0 -2 2 -1 0 -1 2 -2 0 -2 2 -1 0 -3 4 -4 0 -4 4 -3 0", "0 -1 2 -2 0 -2 2 -1 0 -3 4 -4 0 -4 4 -3 0 -1 2 -2 0 -2 2 -1 0", "0 -3 4 -4 0 -4 4 -3 0 -3 4 -4 0 -4 4 -3 0 -1 2 -2 0 -2 2 -1 0", "0 -3 4 -4 0 -4 4 -3 0 -1 2 -2 0 -2 2 -1 0 -3 4 -4 0 -4 4 -3 0", "0 -1 1 -4 0 -4 1 -1 0 -1 1 -4 0 -4 1 -1 0 -3 4 -4 0 -4 4 -3 0", "0 -1 1 -4 0 -4 1 -1 0 -3 4 -4 0 -4 4 -3 0 -1 1 -4 0 -4 1 -1 0", "0 -3 4 -4 0 -4 4 -3 0 -3 4 -4 0 -4 4 -3 0 -1 1 -4 0 -4 1 -1 0", "0 -3 4 -4 0 -4 4 -3 0 -1 1 -4 0 -4 1 -1 0 -3 4 -4 0 -4 4 -3 0", "0 -1 2 -2 0 -2 2 -1 0 -1 2 -2 0 -2 2 -1 0 -2 3 -3 0 -3 3 -2 0", "0 -1 2 -2 0 -2 2 -1 0 -2 3 -3 0 -3 3 -2 0 -1 2 -2 0 -2 2 -1 0", "0 -2 3 -3 0 -3 3 -2 0 -2 3 -3 0 -3 3 -2 0 -1 2 -2 0 -2 2 -1 0", "0 -2 3 -3 0 -3 3 -2 0 -1 2 -2 0 -2 2 -1 0 -2 3 -3 0 -3 3 -2 0"]
  in  "file path (to write) 2":path
  in  "save":bool
  in  "cycles":i32=1
  out "Array 2":string[](array[string])
  in  "cluster centers (original) 5":string[](array[string])=["0 -1 1 -4 0 -4 1 -1 0 -1 1 -4 0 -4 1 -1 0 -1 1 -4 0 -4 1 -1 0 -1 0 -1 1 -4 0 -4 1 -1 0", "0 -1 2 -2 0 -2 2 -1 0 -1 2 -2 0 -2 2 -1 0 -1 2 -2 0 -2 2 -1 0 -1 0 -1 2 -2 0 -2 2 -1 0", "0 -2 3 -3 0 -3 3 -2 0 -2 3 -3 0 -3 3 -2 0 -2 3 -3 0 -3 3 -2 0 -2 0 -2 3 -3 0 -3 3 -2 0", "0 -3 4 -4 0 -4 4 -3 0 -3 4 -4 0 -4 4 -3 0 -3 4 -4 0 -4 4 -3 0 -3 0 -3 4 -4 0 -4 4 -3 0", "0 -1 1 -4 4 -3 0 -3 4 -4 1 -1 0 -1 1 -4 4 -3 0 -3 4 -4 1 -1 0 -1 1 -4 4 -3 0 -3 4 -4 1 -1 0 -1 1 -4 4 -3 0 -3 4 -4 1 -1 0", "0 -1 2 -2 3 -3 0 -3 3 -2 2 -1 0 -1 2 -2 3 -3 0 -3 3 -2 2 -1 0 -1 2 -2 3 -3 0 -3 3 -2 2 -1 0 -1 2 -2 3 -3 0 -3 3 -2 2 -1 0", "0 -4 1 -1 2 -2 0 -2 2 -1 1 -4 0 -4 1 -1 2 -2 0 -2 2 -1 1 -4 0 -4 1 -1 2 -2 0 -2 2 -1 1 -4 0 -4 1 -1 2 -2 0 -2 2 -1 1 -4 0", "0 -4 4 -3 3 -2 0 -2 3 -3 4 -4 0 -4 4 -3 3 -2 0 -2 3 -3 4 -4 0 -4 4 -3 3 -2 0 -2 3 -3 4 -4 0 -4 4 -3 3 -2 0 -2 3 -3 4 -4 0", "0 -1 1 -4 0 -2 3 -3 0 -3 3 -2 0 -4 1 -1 0 -1 1 -4 0 -2 3 -3 0 -3 3 -2 0 -4 1 -1 0 -1 1 -4 0 -2 3 -3 0 -3 3 -2 0 -4 1 -1 0 -1 1 -4 0 -2 3 -3 0 -3 3 -2 0 -4 1 -1 0", "0 -1 2 -2 0 -4 4 -3 0 -3 4 -4 0 -2 2 -1 0 -1 2 -2 0 -4 4 -3 0 -3 4 -4 0 -2 2 -1 0 -1 2 -2 0 -4 4 -3 0 -3 4 -4 0 -2 2 -1 0 -1 2 -2 0 -4 4 -3 0 -3 4 -4 0 -2 2 -1 0"]
  in  "cluster centers (original) 4":string[](array[string])=["0 -1 1 -4 0 -4 1 -1 0 -1 1 -4 0 -4 1 -1 0", "0 -1 2 -2 0 -2 2 -1 0 -1 2 -2 0 -2 2 -1 0", "0 -2 3 -3 0 -3 3 -2 0 -2 3 -3 0 -3 3 -2 0", "0 -3 4 -4 0 -4 4 -3 0 -3 4 -4 0 -4 4 -3 0", "0 -1 1 -4 4 -3 0 -3 4 -4 1 -1 0 -1 1 -4 4 -3 0 -3 4 -4 1 -1 0", "0 -1 2 -2 3 -3 0 -3 3 -2 2 -1 0 -1 2 -2 3 -3 0 -3 3 -2 2 -1 0", "0 -4 1 -1 2 -2 0 -2 2 -1 1 -4 0 -4 1 -1 2 -2 0 -2 2 -1 1 -4 0", "0 -4 4 -3 3 -2 0 -2 3 -3 4 -4 0 -4 4 -3 3 -2 0 -2 3 -3 4 -4 0", "0 -1 1 -4 0 -2 3 -3 0 -3 3 -2 0 -4 1 -1 0 -1 1 -4 0 -2 3 -3 0 -3 3 -2 0 -4 1 -1 0", "0 -1 2 -2 0 -4 4 -3 0 -3 4 -4 0 -2 2 -1 0 -1 2 -2 0 -4 4 -3 0 -3 4 -4 0 -2 2 -1 0"]
  out "size(s)":i32
  in  "cluster centers (original) 3":string[](array[string])=["0 -1 1 -4 0 -4 1 -1 0 -1 1 -4 0 -4 1 -1 0 -1 1 -4 0 -4 1 -1 0", "0 -1 2 -2 0 -2 2 -1 0 -1 2 -2 0 -2 2 -1 0 -1 2 -2 0 -2 2 -1 0", "0 -2 3 -3 0 -3 3 -2 0 -2 3 -3 0 -3 3 -2 0 -2 3 -3 0 -3 3 -2 0", "0 -3 4 -4 0 -4 4 -3 0 -3 4 -4 0 -4 4 -3 0 -3 4 -4 0 -4 4 -3 0", "0 -1 1 -4 4 -3 0 -3 4 -4 1 -1 0 -1 1 -4 4 -3 0 -3 4 -4 1 -1 0 -1 1 -4 4 -3 0 -3 4 -4 1 -1 0", "0 -1 2 -2 3 -3 0 -3 3 -2 2 -1 0 -1 2 -2 3 -3 0 -3 3 -2 2 -1 0 -1 2 -2 3 -3 0 -3 3 -2 2 -1 0", "0 -4 1 -1 2 -2 0 -2 2 -1 1 -4 0 -4 1 -1 2 -2 0 -2 2 -1 1 -4 0 -4 1 -1 2 -2 0 -2 2 -1 1 -4 0", "0 -4 4 -3 3 -2 0 -2 3 -3 4 -4 0 -4 4 -3 3 -2 0 -2 3 -3 4 -4 0 -4 4 -3 3 -2 0 -2 3 -3 4 -4 0", "0 -1 1 -4 0 -2 3 -3 0 -3 3 -2 0 -4 1 -1 0 -1 1 -4 0 -2 3 -3 0 -3 3 -2 0 -4 1 -1 0 -1 1 -4 0 -2 3 -3 0 -3 3 -2 0 -4 1 -1 0", "0 -1 2 -2 0 -4 4 -3 0 -3 4 -4 0 -2 2 -1 0 -1 2 -2 0 -4 4 -3 0 -3 4 -4 0 -2 2 -1 0 -1 2 -2 0 -4 4 -3 0 -3 4 -4 0 -2 2 -1 0"]
  in  "cluster centers (original) 2":string[](array[string])=["0 -1 1 -4 0 -4 1 -1 0", "0 -1 2 -2 0 -2 2 -1 0", "0 -2 3 -3 0 -3 3 -2 0", "0 -3 4 -4 0 -4 4 -3 0", "0 -1 1 -4 4 -3 0 -3 4 -4 1 -1 0", "0 -1 2 -2 3 -3 0 -3 3 -2 2 -1 0", "0 -4 1 -1 2 -2 0 -2 2 -1 1 -4 0", "0 -4 4 -3 3 -2 0 -2 3 -3 4 -4 0", "0 -1 1 -4 0 -2 3 -3 0 -3 3 -2 0 -4 1 -1 0", "0 -1 2 -2 0 -4 4 -3 0 -3 4 -4 0 -2 2 -1 0"]
  out "accuracy":string[][](array[string])
  in  "cluster centers 2 centers for diagonals - long - original clusters 5":string[](array[string])=["1 0 -1 1 -1 0 -4 1 -4 0 1 0 -1 1 -1 0 -4 1 -4 0 1 0 -1 1 -1 0 -4 1 -4 0 1 0 -1 1 -1 0 -4 1 -4 0 1 0 -1 1 -1 0 -4 1 -4 0 1", "2 0 -1 2 -1 0 -2 2 -2 0 2 0 -1 2 -1 0 -2 2 -2 0 2 0 -1 2 -1 0 -2 2 -2 0 2 0 -1 2 -1 0 -2 2 -2 0 2 0 -1 2 -1 0 -2 2 -2 0 2", "3 0 -3 3 -3 0 -2 3 -2 0 3 0 -3 3 -3 0 -2 3 -2 0 3 0 -3 3 -3 0 -2 3 -2 0 3 0 -3 3 -3 0 -2 3 -2 0 3 0 -3 3 -3 0 -2 3 -2 0 3", "4 0 -3 4 -3 0 -4 4 -4 0 4 0 -3 4 -3 0 -4 4 -4 0 4 0 -3 4 -3 0 -4 4 -4 0 4 0 -3 4 -3 0 -4 4 -4 0 4 0 -3 4 -3 0 -4 4 -4 0 4", "-1 1 -4 0 -4 4 -3 4 -4 0 -4 1 -1 1 -4 0 -4 4 -3 4 -4 0 -4 1 -1 1 -4 0 -4 4 -3 4 -4 0 -4 1 -1 1 -4 0 -4 4 -3 4 -4 0 -4 1 -1 1 -4 0 -4 4 -3 4 -4 0 -4 1 -1", "-1 2 -2 0 -2 3 -3 3 -2 0 -2 2 -1 2 -2 0 -2 3 -3 3 -2 0 -2 2 -1 2 -2 0 -2 3 -3 3 -2 0 -2 2 -1 2 -2 0 -2 3 -3 3 -2 0 -2 2 -1 2 -2 0 -2 3 -3 3 -2 0 -2 2 -1", "-4 1 -1 0 -1 2 -2 2 -1 0 -1 1 -4 1 -1 0 -1 2 -2 2 -1 0 -1 1 -4 1 -1 0 -1 2 -2 2 -1 0 -1 1 -4 1 -1 0 -1 2 -2 2 -1 0 -1 1 -4 1 -1 0 -1 2 -2 2 -1 0 -1 1 -4", "-4 4 -3 0 -3 3 -2 3 -3 0 -3 4 -4 4 -3 0 -3 3 -2 3 -3 0 -3 4 -4 4 -3 0 -3 3 -2 3 -3 0 -3 4 -4 4 -3 0 -3 3 -2 3 -3 0 -3 4 -4 4 -3 0 -3 3 -2 3 -3 0 -3 4 -4", "0 1 -1 0 -3 3 0 3 -3 0 -1 1 0 1 -1 0 -3 3 0 3 -3 0 -1 1 0 1 -1 0 -3 3 0 3 -3 0 -1 1 0 1 -1 0 -3 3 0 3 -3 0 -1 1 0 1 -1 0 -3 3 0 3 -3 0 -1 1 0", "0 1 -4 0 -2 3 0 3 -2 0 -4 1 0 1 -4 0 -2 3 0 3 -2 0 -4 1 0 1 -4 0 -2 3 0 3 -2 0 -4 1 0 1 -4 0 -2 3 0 3 -2 0 -4 1 0 1 -4 0 -2 3 0 3 -2 0 -4 1 0", "0 4 -3 0 -1 2 0 2 -1 0 -3 4 0 4 -3 0 -1 2 0 2 -1 0 -3 4 0 4 -3 0 -1 2 0 2 -1 0 -3 4 0 4 -3 0 -1 2 0 2 -1 0 -3 4 0 4 -3 0 -1 2 0 2 -1 0 -3 4 0", "0 4 -4 0 -2 2 0 2 -2 0 -4 4 0 4 -4 0 -2 2 0 2 -2 0 -4 4 0 4 -4 0 -2 2 0 2 -2 0 -4 4 0 4 -4 0 -2 2 0 2 -2 0 -4 4 0 4 -4 0 -2 2 0 2 -2 0 -4 4 0"]
  in  "cluster centers 2 centers for diagonals - long - original clusters 4":string[](array[string])=["1 0 -1 1 -1 0 -4 1 -4 0 1 0 -1 1 -1 0 -4 1 -4 0 1 0 -1 1 -1 0 -4 1 -4 0 1 0 -1 1 -1 0 -4 1 -4 0 1", "2 0 -1 2 -1 0 -2 2 -2 0 2 0 -1 2 -1 0 -2 2 -2 0 2 0 -1 2 -1 0 -2 2 -2 0 2 0 -1 2 -1 0 -2 2 -2 0 2", "3 0 -3 3 -3 0 -2 3 -2 0 3 0 -3 3 -3 0 -2 3 -2 0 3 0 -3 3 -3 0 -2 3 -2 0 3 0 -3 3 -3 0 -2 3 -2 0 3", "4 0 -3 4 -3 0 -4 4 -4 0 4 0 -3 4 -3 0 -4 4 -4 0 4 0 -3 4 -3 0 -4 4 -4 0 4 0 -3 4 -3 0 -4 4 -4 0 4", "-1 1 -4 0 -4 4 -3 4 -4 0 -4 1 -1 1 -4 0 -4 4 -3 4 -4 0 -4 1 -1 1 -4 0 -4 4 -3 4 -4 0 -4 1 -1 1 -4 0 -4 4 -3 4 -4 0 -4 1 -1", "-1 2 -2 0 -2 3 -3 3 -2 0 -2 2 -1 2 -2 0 -2 3 -3 3 -2 0 -2 2 -1 2 -2 0 -2 3 -3 3 -2 0 -2 2 -1 2 -2 0 -2 3 -3 3 -2 0 -2 2 -1", "-4 1 -1 0 -1 2 -2 2 -1 0 -1 1 -4 1 -1 0 -1 2 -2 2 -1 0 -1 1 -4 1 -1 0 -1 2 -2 2 -1 0 -1 1 -4 1 -1 0 -1 2 -2 2 -1 0 -1 1 -4", "-4 4 -3 0 -3 3 -2 3 -3 0 -3 4 -4 4 -3 0 -3 3 -2 3 -3 0 -3 4 -4 4 -3 0 -3 3 -2 3 -3 0 -3 4 -4 4 -3 0 -3 3 -2 3 -3 0 -3 4 -4", "0 1 -1 0 -3 3 0 3 -3 0 -1 1 0 1 -1 0 -3 3 0 3 -3 0 -1 1 0 1 -1 0 -3 3 0 3 -3 0 -1 1 0 1 -1 0 -3 3 0 3 -3 0 -1 1 0", "0 1 -4 0 -2 3 0 3 -2 0 -4 1 0 1 -4 0 -2 3 0 3 -2 0 -4 1 0 1 -4 0 -2 3 0 3 -2 0 -4 1 0 1 -4 0 -2 3 0 3 -2 0 -4 1 0", "0 4 -3 0 -1 2 0 2 -1 0 -3 4 0 4 -3 0 -1 2 0 2 -1 0 -3 4 0 4 -3 0 -1 2 0 2 -1 0 -3 4 0 4 -3 0 -1 2 0 2 -1 0 -3 4 0", "0 4 -4 0 -2 2 0 2 -2 0 -4 4 0 4 -4 0 -2 2 0 2 -2 0 -4 4 0 4 -4 0 -2 2 0 2 -2 0 -4 4 0 4 -4 0 -2 2 0 2 -2 0 -4 4 0"]
  in  "cluster centers 2 centers for diagonals - long - original clusters 3":string[](array[string])=["1 0 -1 1 -1 0 -4 1 -4 0 1 0 -1 1 -1 0 -4 1 -4 0 1 0 -1 1 -1 0 -4 1 -4 0 1", "2 0 -1 2 -1 0 -2 2 -2 0 2 0 -1 2 -1 0 -2 2 -2 0 2 0 -1 2 -1 0 -2 2 -2 0 2", "3 0 -3 3 -3 0 -2 3 -2 0 3 0 -3 3 -3 0 -2 3 -2 0 3 0 -3 3 -3 0 -2 3 -2 0 3", "4 0 -3 4 -3 0 -4 4 -4 0 4 0 -3 4 -3 0 -4 4 -4 0 4 0 -3 4 -3 0 -4 4 -4 0 4", "-1 1 -4 0 -4 4 -3 4 -4 0 -4 1 -1 1 -4 0 -4 4 -3 4 -4 0 -4 1 -1 1 -4 0 -4 4 -3 4 -4 0 -4 1 -1", "-1 2 -2 0 -2 3 -3 3 -2 0 -2 2 -1 2 -2 0 -2 3 -3 3 -2 0 -2 2 -1 2 -2 0 -2 3 -3 3 -2 0 -2 2 -1", "-4 1 -1 0 -1 2 -2 2 -1 0 -1 1 -4 1 -1 0 -1 2 -2 2 -1 0 -1 1 -4 1 -1 0 -1 2 -2 2 -1 0 -1 1 -4", "-4 4 -3 0 -3 3 -2 3 -3 0 -3 4 -4 4 -3 0 -3 3 -2 3 -3 0 -3 4 -4 4 -3 0 -3 3 -2 3 -3 0 -3 4 -4", "0 1 -1 0 -3 3 0 3 -3 0 -1 1 0 1 -1 0 -3 3 0 3 -3 0 -1 1 0 1 -1 0 -3 3 0 3 -3 0 -1 1 0", "0 1 -4 0 -2 3 0 3 -2 0 -4 1 0 1 -4 0 -2 3 0 3 -2 0 -4 1 0 1 -4 0 -2 3 0 3 -2 0 -4 1 0", "0 4 -3 0 -1 2 0 2 -1 0 -3 4 0 4 -3 0 -1 2 0 2 -1 0 -3 4 0 4 -3 0 -1 2 0 2 -1 0 -3 4 0", "0 4 -4 0 -2 2 0 2 -2 0 -4 4 0 4 -4 0 -2 2 0 2 -2 0 -4 4 0 4 -4 0 -2 2 0 2 -2 0 -4 4 0"]
  in  "cluster centers 2 centers for diagonals - short - original clusters":string[](array[string])=["1 0 -1 1 -1 0 -4 1 -4 0 1", "2 0 -1 2 -1 0 -2 2 -2 0 2", "3 0 -3 3 -3 0 -2 3 -2 0 3", "4 0 -3 4 -3 0 -4 4 -4 0 4", "-1 1 -4 0 -4 4 -3 4 -4 0 -4 1 -1", "-1 2 -2 0 -2 3 -3 3 -2 0 -2 2 -1", "-4 1 -1 0 -1 2 -2 2 -1 0 -1 1 -4", "-4 4 -3 0 -3 3 -2 3 -3 0 -3 4 -4", "0 1 -1 0 -3 3 0 3 -3 0 -1 1 0", "0 1 -4 0 -2 3 0 3 -2 0 -4 1 0", "0 4 -3 0 -1 2 0 2 -1 0 -3 4 0", "0 4 -4 0 -2 2 0 2 -2 0 -4 4 0"]
  in  "cluster centers 2 centers for diagonals - long - original clusters":string[](array[string])=["1 0 -1 1 -1 0 -4 1 -4 0 1 0 -1 1 -1 0 -4 1 -4 0 1", "2 0 -1 2 -1 0 -2 2 -2 0 2 0 -1 2 -1 0 -2 2 -2 0 2", "3 0 -3 3 -3 0 -2 3 -2 0 3 0 -3 3 -3 0 -2 3 -2 0 3", "4 0 -3 4 -3 0 -4 4 -4 0 4 0 -3 4 -3 0 -4 4 -4 0 4", "-1 1 -4 0 -4 4 -3 4 -4 0 -4 1 -1 1 -4 0 -4 4 -3 4 -4 0 -4 1 -1", "-1 2 -2 0 -2 3 -3 3 -2 0 -2 2 -1 2 -2 0 -2 3 -3 3 -2 0 -2 2 -1", "-4 1 -1 0 -1 2 -2 2 -1 0 -1 1 -4 1 -1 0 -1 2 -2 2 -1 0 -1 1 -4", "-4 4 -3 0 -3 3 -2 3 -3 0 -3 4 -4 4 -3 0 -3 3 -2 3 -3 0 -3 4 -4", "0 1 -1 0 -3 3 0 3 -3 0 -1 1 0 1 -1 0 -3 3 0 3 -3 0 -1 1 0", "0 1 -4 0 -2 3 0 3 -2 0 -4 1 0 1 -4 0 -2 3 0 3 -2 0 -4 1 0", "0 4 -3 0 -1 2 0 2 -1 0 -3 4 0 4 -3 0 -1 2 0 2 -1 0 -3 4 0", "0 4 -4 0 -2 2 0 2 -2 0 -4 4 0 4 -4 0 -2 2 0 2 -2 0 -4 4 0"]
  in  "cluster centers (original) long 5":string[](array[string])=["1 0 -1 1 -1 0 -4 1 -4 0 1 0 -1 1 -1 0 -4 1 -4 0 1 0 -1 1 -1 0 -4 1 -4 0 1 0 -1 1 -1 0 -4 1 -4 0 1 0 -1 1 -1 0 -4 1 -4 0 1", "2 0 -1 2 -1 0 -2 2 -2 0 2 0 -1 2 -1 0 -2 2 -2 0 2 0 -1 2 -1 0 -2 2 -2 0 2 0 -1 2 -1 0 -2 2 -2 0 2 0 -1 2 -1 0 -2 2 -2 0 2", "3 0 -3 3 -3 0 -2 3 -2 0 3 0 -3 3 -3 0 -2 3 -2 0 3 0 -3 3 -3 0 -2 3 -2 0 3 0 -3 3 -3 0 -2 3 -2 0 3 0 -3 3 -3 0 -2 3 -2 0 3", "4 0 -3 4 -3 0 -4 4 -4 0 4 0 -3 4 -3 0 -4 4 -4 0 4 0 -3 4 -3 0 -4 4 -4 0 4 0 -3 4 -3 0 -4 4 -4 0 4 0 -3 4 -3 0 -4 4 -4 0 4", "-1 1 -4 0 -4 4 -3 4 -4 0 -4 1 -1 1 -4 0 -4 4 -3 4 -4 0 -4 1 -1 1 -4 0 -4 4 -3 4 -4 0 -4 1 -1 1 -4 0 -4 4 -3 4 -4 0 -4 1 -1 1 -4 0 -4 4 -3 4 -4 0 -4 1 -1", "-1 2 -2 0 -2 3 -3 3 -2 0 -2 2 -1 2 -2 0 -2 3 -3 3 -2 0 -2 2 -1 2 -2 0 -2 3 -3 3 -2 0 -2 2 -1 2 -2 0 -2 3 -3 3 -2 0 -2 2 -1 2 -2 0 -2 3 -3 3 -2 0 -2 2 -1", "-4 1 -1 0 -1 2 -2 2 -1 0 -1 1 -4 1 -1 0 -1 2 -2 2 -1 0 -1 1 -4 1 -1 0 -1 2 -2 2 -1 0 -1 1 -4 1 -1 0 -1 2 -2 2 -1 0 -1 1 -4 1 -1 0 -1 2 -2 2 -1 0 -1 1 -4", "-4 4 -3 0 -3 3 -2 3 -3 0 -3 4 -4 4 -3 0 -3 3 -2 3 -3 0 -3 4 -4 4 -3 0 -3 3 -2 3 -3 0 -3 4 -4 4 -3 0 -3 3 -2 3 -3 0 -3 4 -4 4 -3 0 -3 3 -2 3 -3 0 -3 4 -4", "0 -4 1 -1 0 -3 3 -2 3 -3 0 -1 1 -4 0 -4 1 -1 0 -3 3 -2 3 -3 0 -1 1 -4 0 -4 1 -1 0 -3 3 -2 3 -3 0 -1 1 -4 0 -4 1 -1 0 -3 3 -2 3 -3 0 -1 1 -4 0 -4 1 -1 0 -3 3 -2 3 -3 0 -1 1 -4 0", "0 -4 4 -3 0 -1 2 -2 2 -1 0 -3 4 -4 0 -4 4 -3 0 -1 2 -2 2 -1 0 -3 4 -4 0 -4 4 -3 0 -1 2 -2 2 -1 0 -3 4 -4 0 -4 4 -3 0 -1 2 -2 2 -1 0 -3 4 -4 0 -4 4 -3 0 -1 2 -2 2 -1 0 -3 4 -4 0"]
  in  "cluster centers (original) long 4":string[](array[string])=["1 0 -1 1 -1 0 -4 1 -4 0 1 0 -1 1 -1 0 -4 1 -4 0 1 0 -1 1 -1 0 -4 1 -4 0 1 0 -1 1 -1 0 -4 1 -4 0 1", "2 0 -1 2 -1 0 -2 2 -2 0 2 0 -1 2 -1 0 -2 2 -2 0 2 0 -1 2 -1 0 -2 2 -2 0 2 0 -1 2 -1 0 -2 2 -2 0 2", "3 0 -3 3 -3 0 -2 3 -2 0 3 0 -3 3 -3 0 -2 3 -2 0 3 0 -3 3 -3 0 -2 3 -2 0 3 0 -3 3 -3 0 -2 3 -2 0 3", "4 0 -3 4 -3 0 -4 4 -4 0 4 0 -3 4 -3 0 -4 4 -4 0 4 0 -3 4 -3 0 -4 4 -4 0 4 0 -3 4 -3 0 -4 4 -4 0 4", "-1 1 -4 0 -4 4 -3 4 -4 0 -4 1 -1 1 -4 0 -4 4 -3 4 -4 0 -4 1 -1 1 -4 0 -4 4 -3 4 -4 0 -4 1 -1 1 -4 0 -4 4 -3 4 -4 0 -4 1 -1", "-1 2 -2 0 -2 3 -3 3 -2 0 -2 2 -1 2 -2 0 -2 3 -3 3 -2 0 -2 2 -1 2 -2 0 -2 3 -3 3 -2 0 -2 2 -1 2 -2 0 -2 3 -3 3 -2 0 -2 2 -1", "-4 1 -1 0 -1 2 -2 2 -1 0 -1 1 -4 1 -1 0 -1 2 -2 2 -1 0 -1 1 -4 1 -1 0 -1 2 -2 2 -1 0 -1 1 -4 1 -1 0 -1 2 -2 2 -1 0 -1 1 -4", "-4 4 -3 0 -3 3 -2 3 -3 0 -3 4 -4 4 -3 0 -3 3 -2 3 -3 0 -3 4 -4 4 -3 0 -3 3 -2 3 -3 0 -3 4 -4 4 -3 0 -3 3 -2 3 -3 0 -3 4 -4", "0 -4 1 -1 0 -3 3 -2 3 -3 0 -1 1 -4 0 -4 1 -1 0 -3 3 -2 3 -3 0 -1 1 -4 0 -4 1 -1 0 -3 3 -2 3 -3 0 -1 1 -4 0 -4 1 -1 0 -3 3 -2 3 -3 0 -1 1 -4 0", "0 -4 4 -3 0 -1 2 -2 2 -1 0 -3 4 -4 0 -4 4 -3 0 -1 2 -2 2 -1 0 -3 4 -4 0 -4 4 -3 0 -1 2 -2 2 -1 0 -3 4 -4 0 -4 4 -3 0 -1 2 -2 2 -1 0 -3 4 -4 0"]
  in  "cluster centers (original) long 3":string[](array[string])=["1 0 -1 1 -1 0 -4 1 -4 0 1 0 -1 1 -1 0 -4 1 -4 0 1 0 -1 1 -1 0 -4 1 -4 0 1", "2 0 -1 2 -1 0 -2 2 -2 0 2 0 -1 2 -1 0 -2 2 -2 0 2 0 -1 2 -1 0 -2 2 -2 0 2", "3 0 -3 3 -3 0 -2 3 -2 0 3 0 -3 3 -3 0 -2 3 -2 0 3 0 -3 3 -3 0 -2 3 -2 0 3", "4 0 -3 4 -3 0 -4 4 -4 0 4 0 -3 4 -3 0 -4 4 -4 0 4 0 -3 4 -3 0 -4 4 -4 0 4", "-1 1 -4 0 -4 4 -3 4 -4 0 -4 1 -1 1 -4 0 -4 4 -3 4 -4 0 -4 1 -1 1 -4 0 -4 4 -3 4 -4 0 -4 1 -1", "-1 2 -2 0 -2 3 -3 3 -2 0 -2 2 -1 2 -2 0 -2 3 -3 3 -2 0 -2 2 -1 2 -2 0 -2 3 -3 3 -2 0 -2 2 -1", "-4 1 -1 0 -1 2 -2 2 -1 0 -1 1 -4 1 -1 0 -1 2 -2 2 -1 0 -1 1 -4 1 -1 0 -1 2 -2 2 -1 0 -1 1 -4", "-4 4 -3 0 -3 3 -2 3 -3 0 -3 4 -4 4 -3 0 -3 3 -2 3 -3 0 -3 4 -4 4 -3 0 -3 3 -2 3 -3 0 -3 4 -4", "0 -4 1 -1 0 -3 3 -2 3 -3 0 -1 1 -4 0 -4 1 -1 0 -3 3 -2 3 -3 0 -1 1 -4 0 -4 1 -1 0 -3 3 -2 3 -3 0 -1 1 -4 0", "0 -4 4 -3 0 -1 2 -2 2 -1 0 -3 4 -4 0 -4 4 -3 0 -1 2 -2 2 -1 0 -3 4 -4 0 -4 4 -3 0 -1 2 -2 2 -1 0 -3 4 -4 0"]
  in  "cluster centers (original) long":string[](array[string])=["1 0 -1 1 -1 0 -4 1 -4 0 1 0 -1 1 -1 0 -4 1 -4 0 1", "2 0 -1 2 -1 0 -2 2 -2 0 2 0 -1 2 -1 0 -2 2 -2 0 2", "3 0 -3 3 -3 0 -2 3 -2 0 3 0 -3 3 -3 0 -2 3 -2 0 3", "4 0 -3 4 -3 0 -4 4 -4 0 4 0 -3 4 -3 0 -4 4 -4 0 4", "-1 1 -4 0 -4 4 -3 4 -4 0 -4 1 -1 1 -4 0 -4 4 -3 4 -4 0 -4 1 -1", "-1 2 -2 0 -2 3 -3 3 -2 0 -2 2 -1 2 -2 0 -2 3 -3 3 -2 0 -2 2 -1", "-4 1 -1 0 -1 2 -2 2 -1 0 -1 1 -4 1 -1 0 -1 2 -2 2 -1 0 -1 1 -4", "-4 4 -3 0 -3 3 -2 3 -3 0 -3 4 -4 4 -3 0 -3 3 -2 3 -3 0 -3 4 -4", "0 -4 1 -1 0 -3 3 -2 3 -3 0 -1 1 -4 0 -4 1 -1 0 -3 3 -2 3 -3 0 -1 1 -4 0", "0 -4 4 -3 0 -1 2 -2 2 -1 0 -3 4 -4 0 -4 4 -3 0 -1 2 -2 2 -1 0 -3 4 -4 0"]
  out "Results":string[][](array[string])
  in  "file path (dialog if empty)":path=path "K:/PhD work/PhD research work 2/Common substring validation/documentation/Data final results/Common substrings (ground truth 2 CHECKED).txt"
  in  "cluster centers (original)":string[](array[string])=["1 0 -1 1 -1 0 -4 1 -4 0 1", "2 0 -1 2 -1 0 -2 2 -2 0 2", "3 0 -3 3 -3 0 -2 3 -2 0 3", "4 0 -3 4 -3 0 -4 4 -4 0 4", "-1 1 -4 0 -4 4 -3 4 -4 0 -4 1 -1", "-1 2 -2 0 -2 3 -3 3 -2 0 -2 2 -1", "-4 1 -1 0 -1 2 -2 2 -1 0 -1 1 -4", "-4 4 -3 0 -3 3 -2 3 -3 0 -3 4 -4", "0 -4 1 -1 0 -3 3 -2 3 -3 0 -1 1 -4 0", "0 -4 4 -3 0 -1 2 -2 2 -1 0 -3 4 -4 0"]
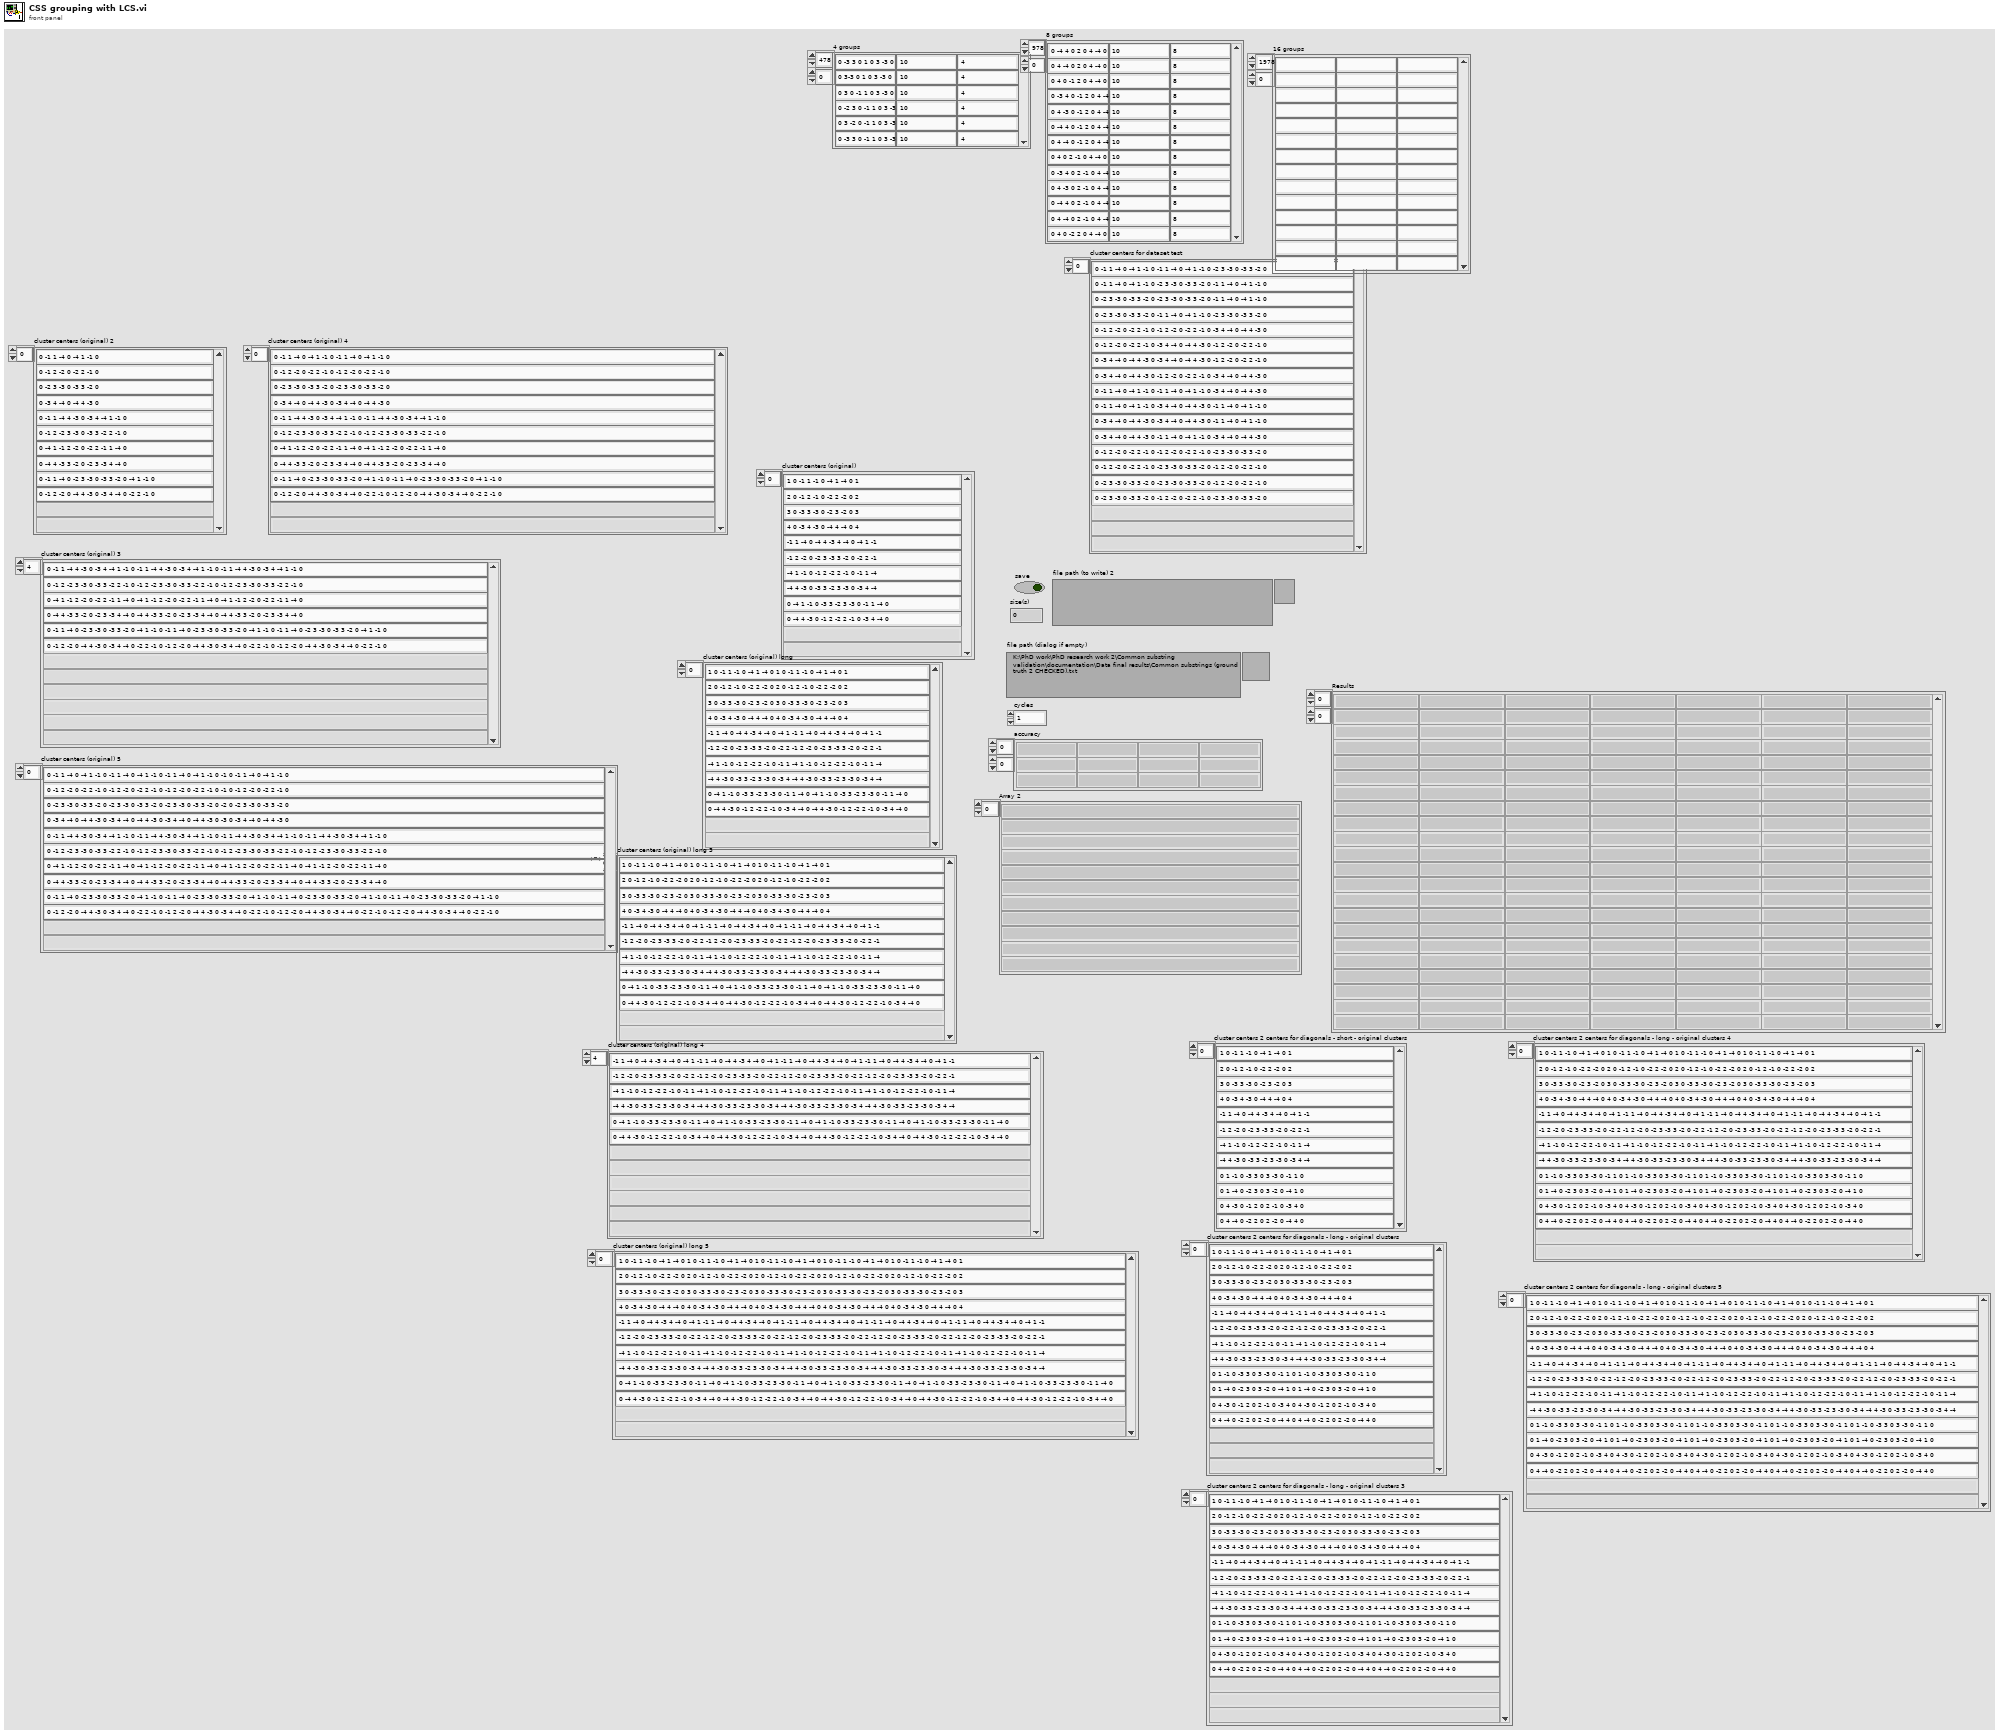
[diagram p1: front panel]
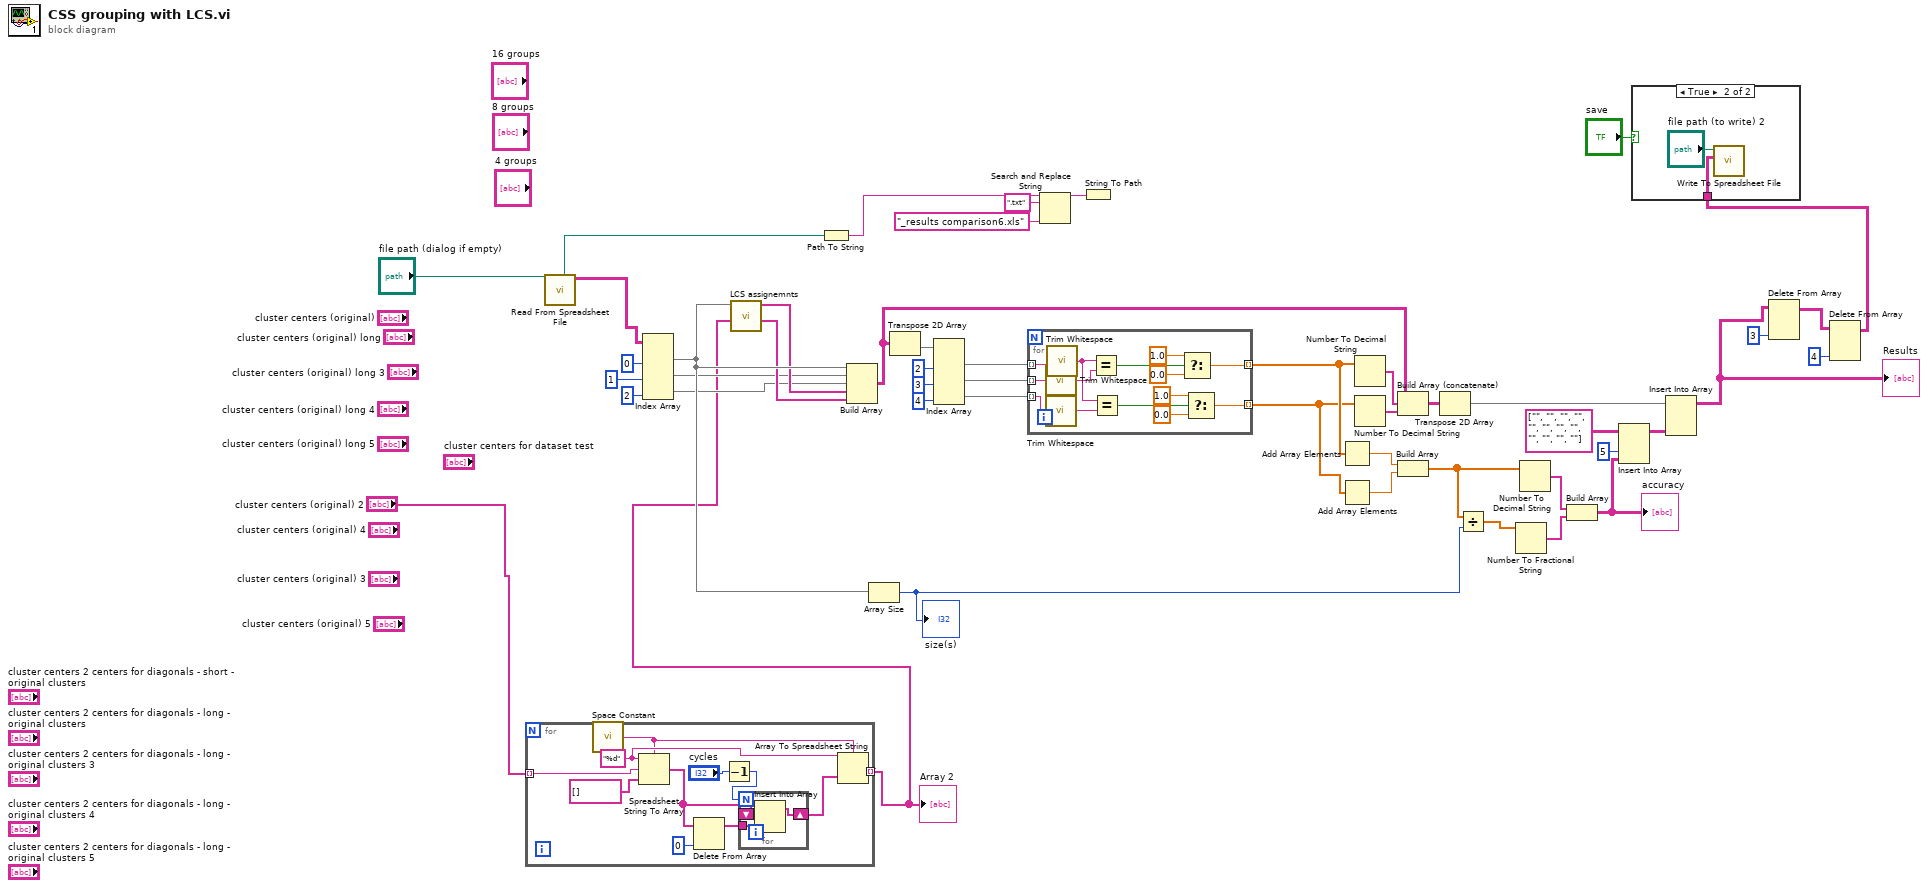
[diagram p0: block diagram]
diagram:
  n1 = for {
    tunnel: "cluster centers (original) 2" -> [w58] mode=indexing
    tunnel: [w54] -> w9 mode=indexing
    w55 = "%d" ("format string")
    n2 = call <vilib>:"Space Constant.vi"() -> ("String"=w53:string)
    n3 = Spreadsheet String To Array(delimiter (Tab)=w53, format string=w55, spreadsheet string=w58, array type (2D Dbl)=string[] []) -> (array=w50:string[])
    n4 = Delete From Array(array=w50, index=0) -> (array with subset deleted=w49:string[])  [unwired: 1 in, 1 out]
    n5 = Decrement(x="cycles") -> (x-1=w52:i32)
    n6 = for {
      N: w52 -> [_]
      tunnel: w49 -> [w61]
      shift-right: [w60] -> w56
      shift-left: w50 -> [w62]
      n7 = Insert Into Array(array=w62, new element=w61) -> (w60:string[])  [unwired: 1 in]
    }
    n8 = Array To Spreadsheet String(delimiter (Tab)=w53, array=w56, 3:w55) -> (spreadsheet string=w54:string)
  }
  "Array 2" <- w9
  n9 = call-poly <vilib>:"Read From Spreadsheet File.vi"("file path (dialog if empty)"="file path (dialog if empty)") -> ("all rows"=w2:string[][], "new file path (Not A Path if cancelled)"=w46:path)  [unwired: 6 in, 3 out]
  n10 = Index Array(array=w2, index (col) #1=0 ("disabled index (col)"), index (col) #2=1 ("index (col)"), index (col) #3=2 ("index (col)")) -> (element #1=w14:string[], element #2=w11:string[], element #3=w10:string[])  [unwired: 3 in]
  n11 = call "LCS assignemnts.vi"("cluster centers"=w9, "Patterns in"=w14) -> ("Assignment (enhanced)"=w12:string[], "Assigned LCS"=w13:string[])  [unwired: 1 in, 7 out]
  n12 = Path To String(path=w46) -> (string=w45:string)
  n13 = Build Array(w14, w11, w10, w13, w12) -> (w31:string[][])
  n14 = Array Size(array=w14) -> (size(s)=w15:i32)
  "size(s)" <- w15
  n15 = Transpose 2D Array(2D array=w31) -> (transposed array=w34:string[][])
  n16 = Index Array(array=w34, index (col) #1=2 ("disabled index (col)"), index (col) #2=3 ("index (col)"), index (col) #3=4 ("index (col)")) -> (element #1=w37:string[], element #2=w36:string[], element #3=w35:string[])  [unwired: 3 in]
  n17 = for {
    tunnel: w37 -> [w68] mode=indexing
    tunnel: w36 -> [w67] mode=indexing
    tunnel: w35 -> [w66] mode=indexing
    tunnel: [w70] -> w18 mode=indexing
    tunnel: [w69] -> w17 mode=indexing
    n18 = call <vilib>:"Trim Whitespace.vi"("string"=w67) -> ("trimmed string"=w65:string)  [unwired: 1 in]
    n19 = call <vilib>:"Trim Whitespace.vi"("string"=w66) -> ("trimmed string"=w64:string)  [unwired: 1 in]
    n20 = call <vilib>:"Trim Whitespace.vi"("string"=w68) -> ("trimmed string"=w63:string)  [unwired: 1 in]
    n21 = Equal?(x=w63, y=w65) -> (x = y?=w76:bool)
    n22 = Equal?(x=w63, y=w64) -> (x = y?=w71:bool)
    n23 = Select(t=1.0, s=w76, f=0.0) -> (s? t:f=w70:dbl)
    n24 = Select(t=1.0, s=w71, f=0.0) -> (s? t:f=w69:dbl)
  }
  n25 = Search and Replace String(input string=w45, search string=".txt", replace string="_results comparison6.xls" ("replace string (\"\")")) -> (result string=w42:string)  [unwired: 5 in, 3 out]
  n26 = String To Path(string=w42) -> ()  [unwired: 1 out]
  n27 = Add Array Elements(numeric array=w18) -> (sum=w19:dbl)
  n28 = Add Array Elements(numeric array=w17) -> (sum=w20:dbl)
  n29 = Number To Decimal String(number=w18) -> (decimal integer string=w33:string[])  [unwired: 1 in]
  n30 = Number To Decimal String(number=w17) -> (decimal integer string=w32:string[])  [unwired: 1 in]
  n31 = Build Array (concatenate)(w31, w33, w32) -> (w30:string[][])
  n32 = Build Array(w19, w20) -> (w21:dbl[])
  n33 = Transpose 2D Array(2D array=w30) -> (transposed array=w16:string[][])
  n34 = Divide(x=w21, y=w15) -> (x/y=w22:dbl[])
  n35 = Number To Fractional String(number=w22) -> (F-format string=w24:string[])  [unwired: 3 in]
  n36 = Number To Decimal String(number=w21) -> (decimal integer string=w23:string[])  [unwired: 1 in]
  n37 = Build Array(w23, w24) -> (w28:string[][])
  "accuracy" <- w28
  n38 = Insert Into Array(array=string[][] [["", "", "", "", "", ""], ["", "", "", "", "", ""]] ("appended array 3"), index (col)=5 ("disabled index (col)"), new element=w28) -> (w27:string[][])  [unwired: 1 in]
  n39 = Insert Into Array(array=w16, new element=w27) -> (w3:string[][])  [unwired: 2 in]
  "Results" <- w3
  n40 = Delete From Array(array=w3, index (col)=3 ("disabled index (col)")) -> (array with subset deleted=w5:string[][])  [unwired: 2 in, 1 out]
  n41 = Delete From Array(array=w5, index (col)=4 ("disabled index (col)")) -> (array with subset deleted=w4:string[][])  [unwired: 2 in, 1 out]
  n42 = case shown="True" "save" {
    tunnel: w4 -> [_ w77]
    frame False {
    }
    frame True {
      n43 = call-poly <vilib>:"Write To Spreadsheet File.vi"("2D data"=w77, "file path (dialog if empty)"="file path (to write) 2") -> ()  [unwired: 6 in, 1 out]
    }
  }
